vi "Condition _string_FOR_Year.vi"(0 "Select Line 2":string(combo)="ST 1", 1 "connection reference":T1, 2 "Shift":string(combo)="ALL", 3 "BREAKDOWN_STK_HOLD_ID":i32=1, 4 "Found Date":string[](array[string]), 5 "year":string(combo)="ST 1", 7 "error in (no error)":errorcluster) -> (12 "Duration count":string[][](array[string]), 13 "error out":errorcluster, 15 "connection reference 2":T1, 18 "BD Count":string[][](array[string]))   [LabVIEW 2017]
uses:
  <vilib>/addons/database/Connection.llb/Conn ObjectReference.ctl
  <vilib>/addons/database/NI_Database_API.lvlib
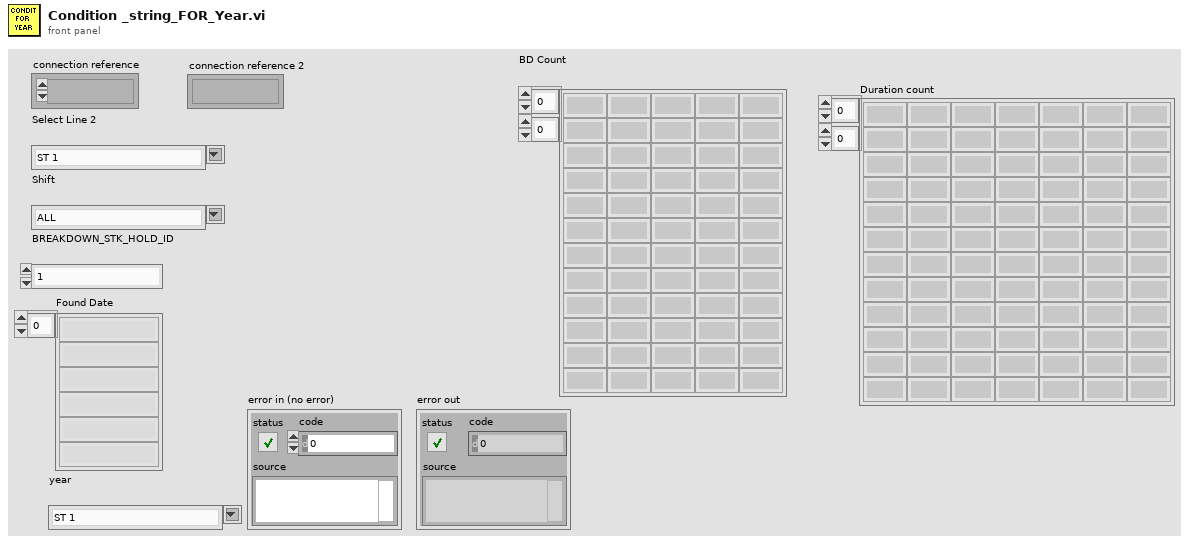
[diagram p1: front panel]
types:
  T1 = typedef "NI_Database_API.lvlib/Conn ObjectReference.ctl" = refnum<k1>
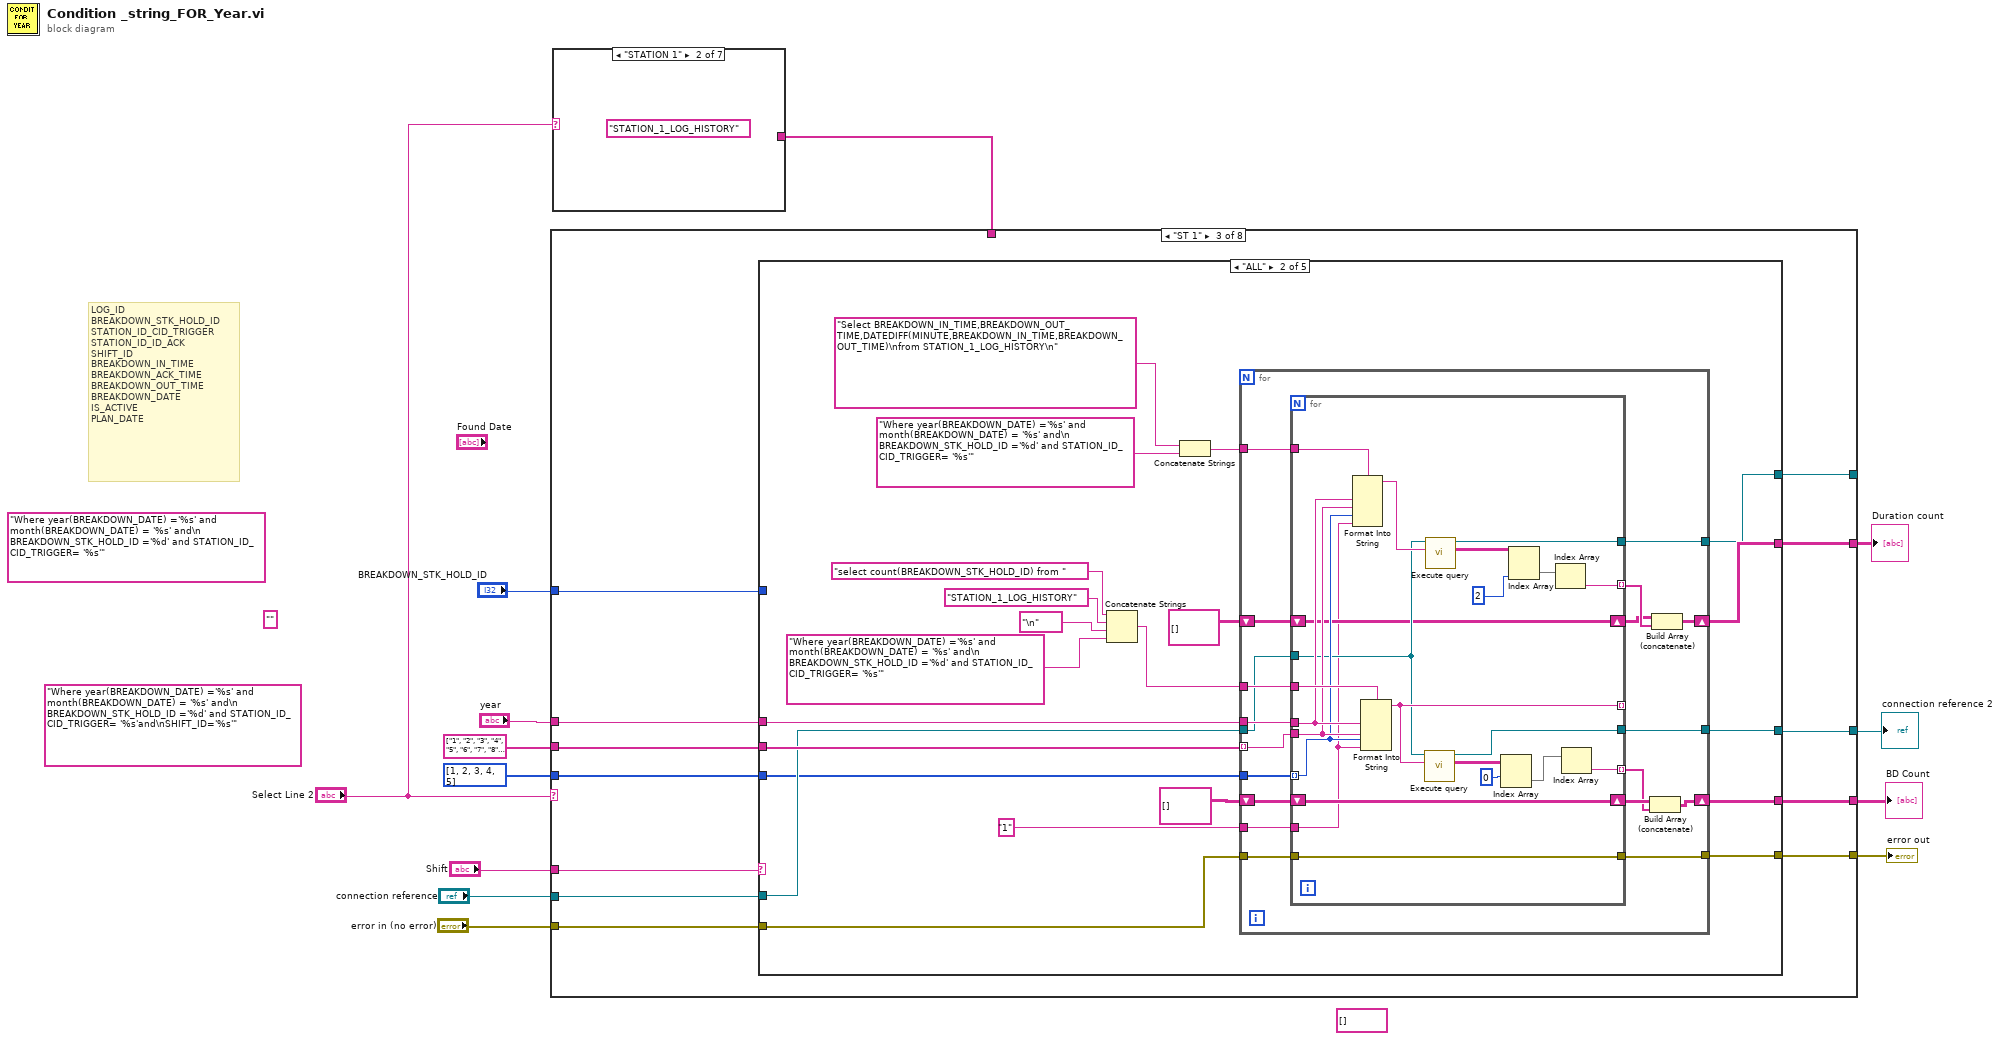
[diagram p0: block diagram]
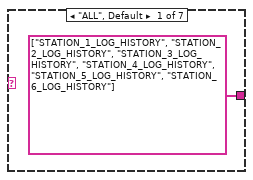
[diagram p2: hidden frame]
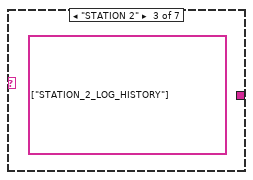
[diagram p3: hidden frame]
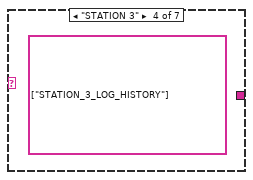
[diagram p4: hidden frame]
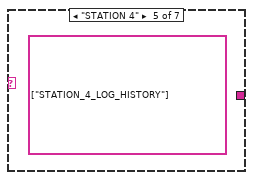
[diagram p5: hidden frame]
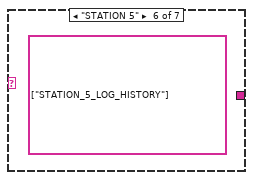
[diagram p6: hidden frame]
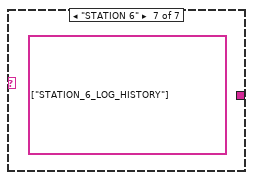
[diagram p7: hidden frame]
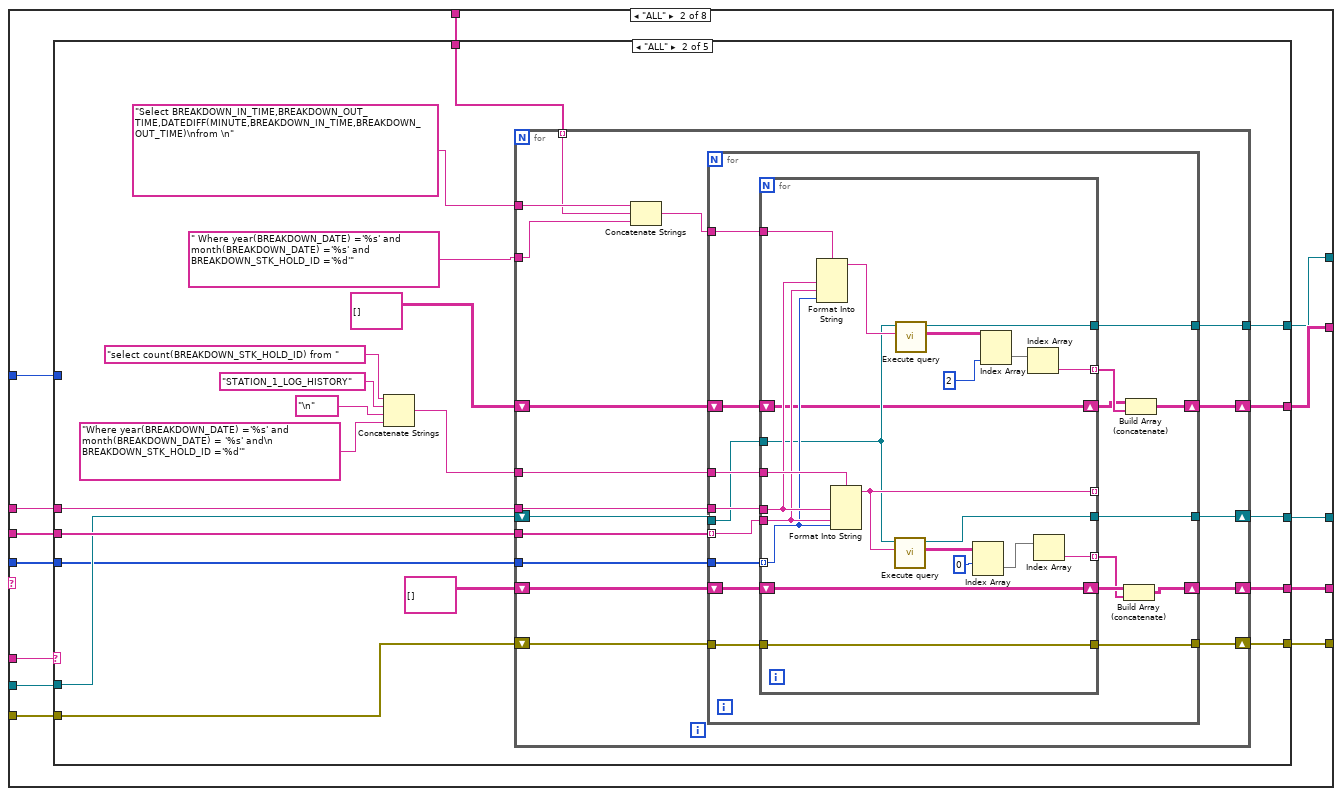
[diagram p9: hidden frame]
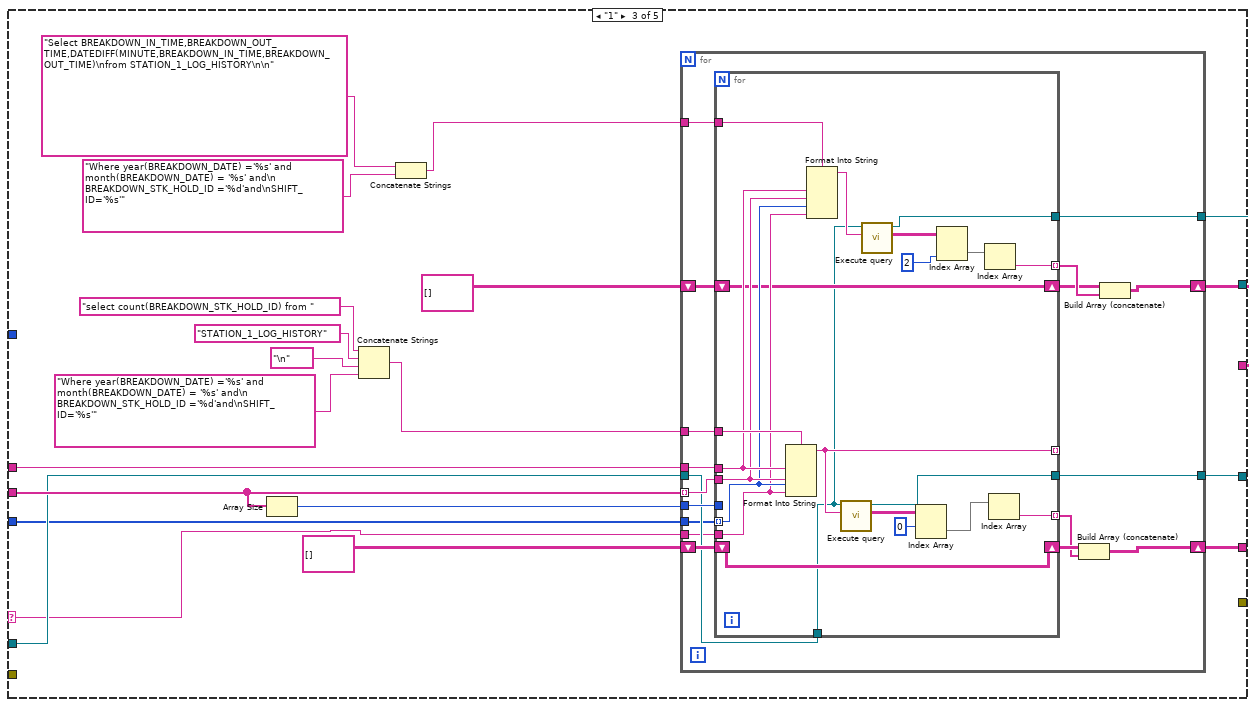
[diagram p11: hidden frame]
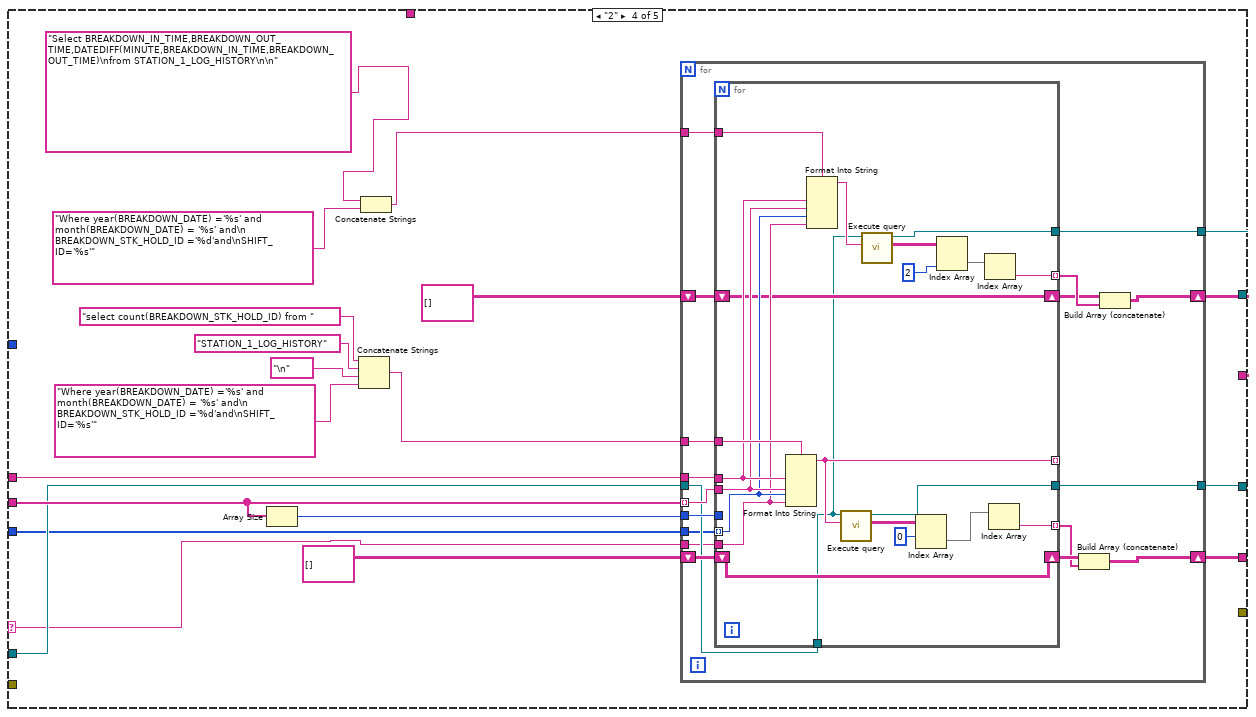
[diagram p12: hidden frame]
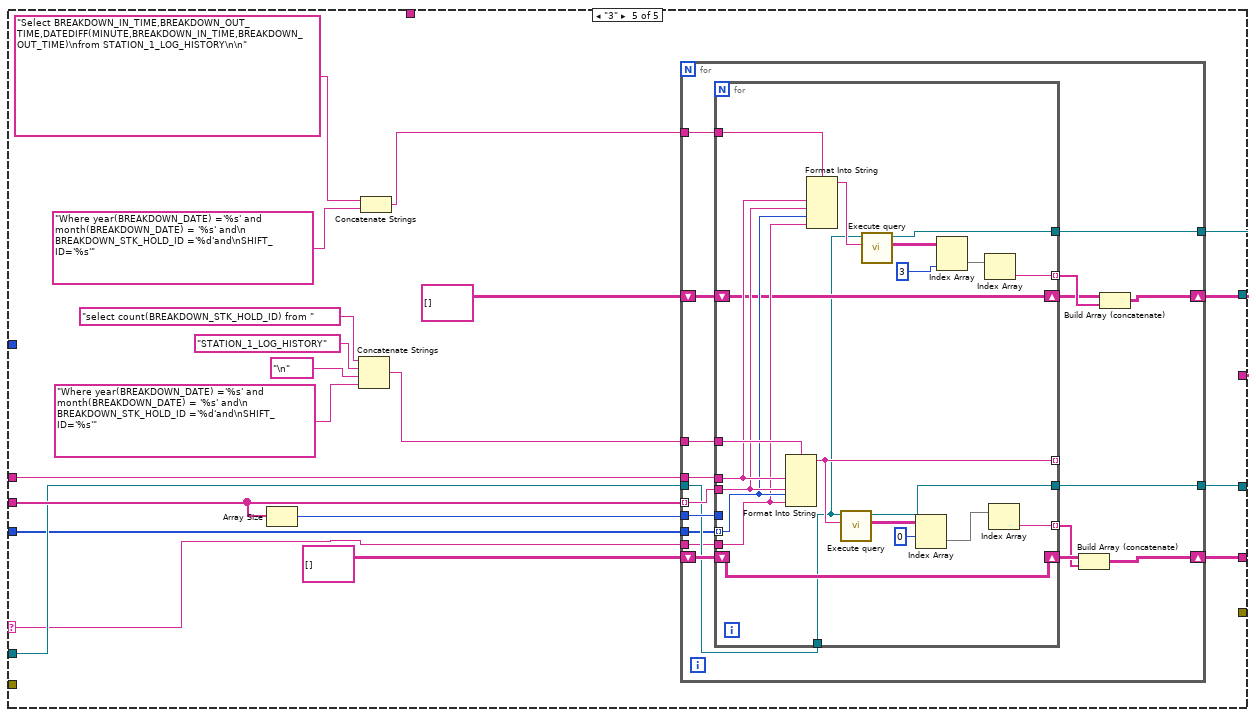
[diagram p13: hidden frame]
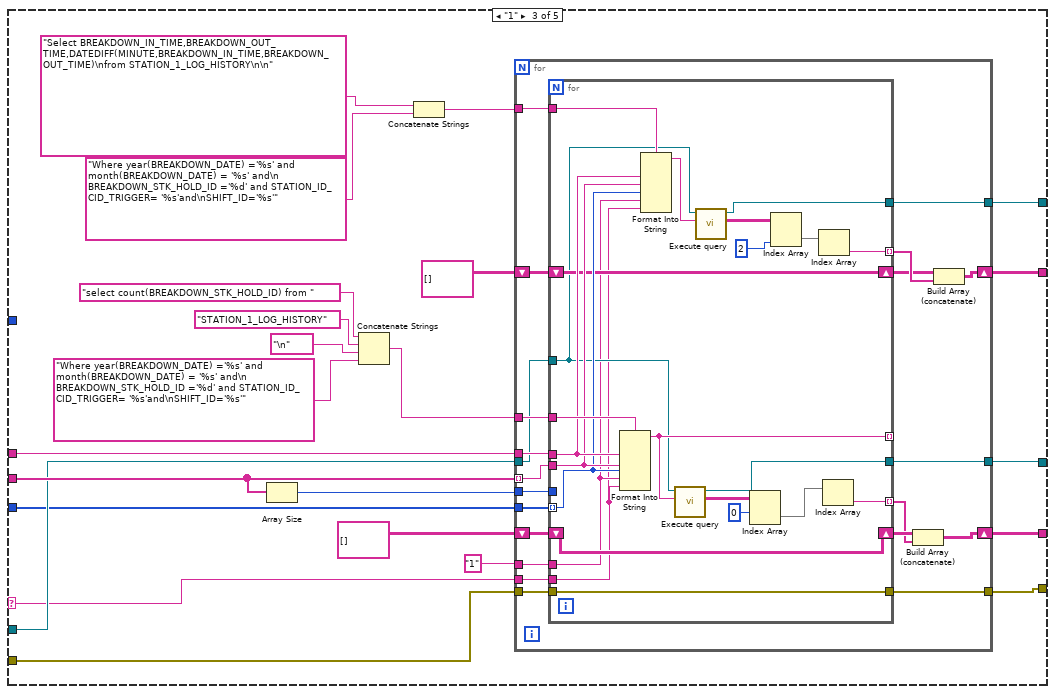
[diagram p15: hidden frame]
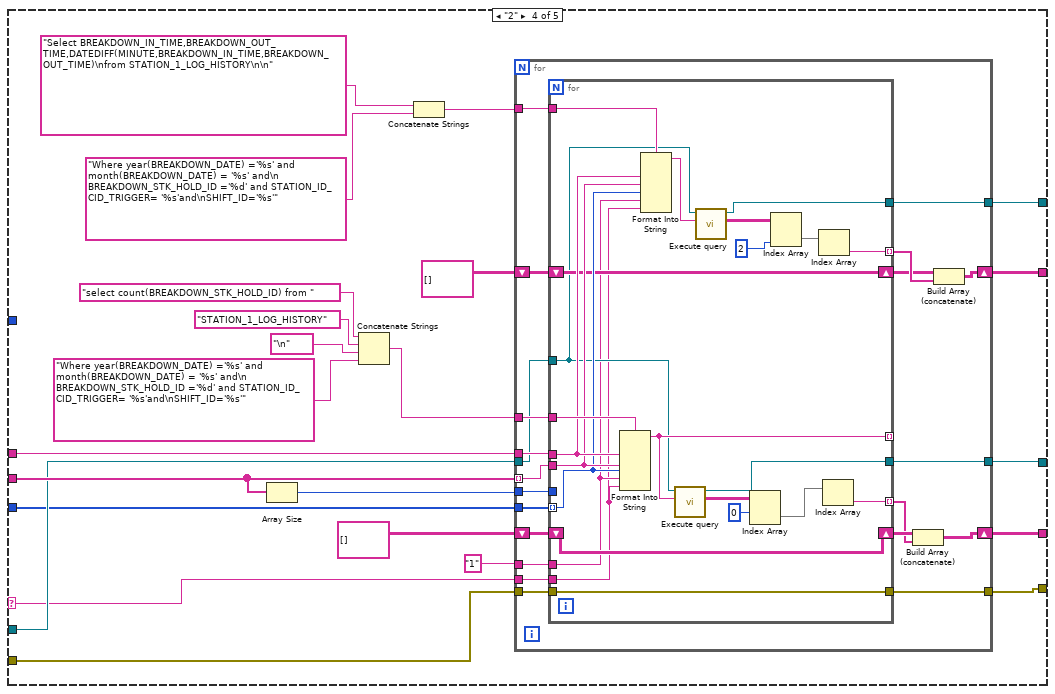
[diagram p16: hidden frame]
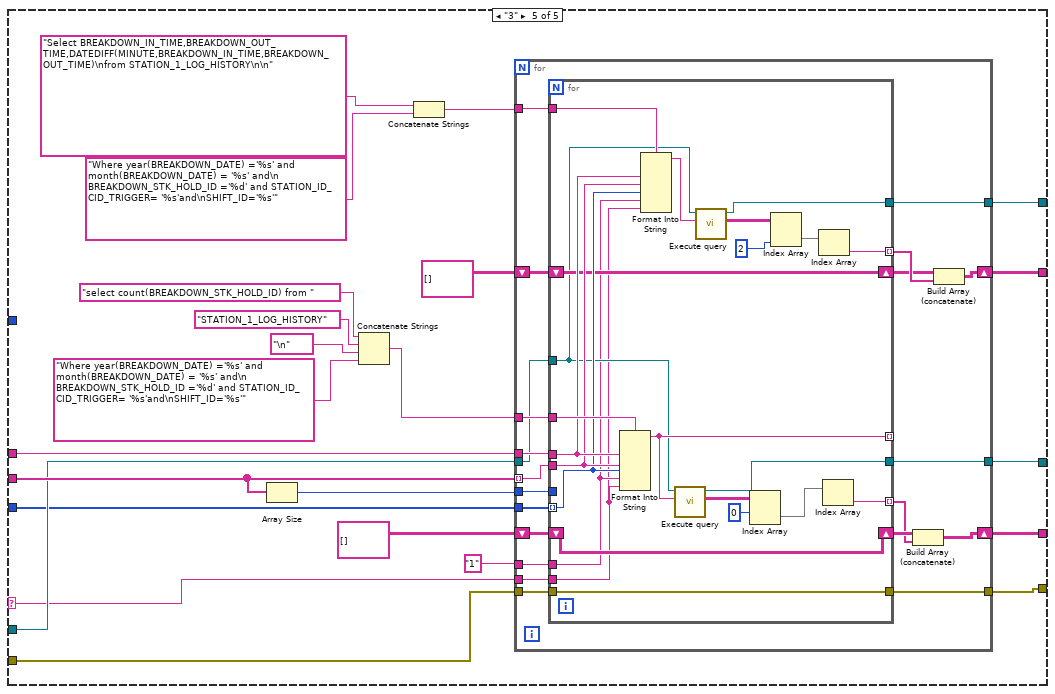
[diagram p17: hidden frame]
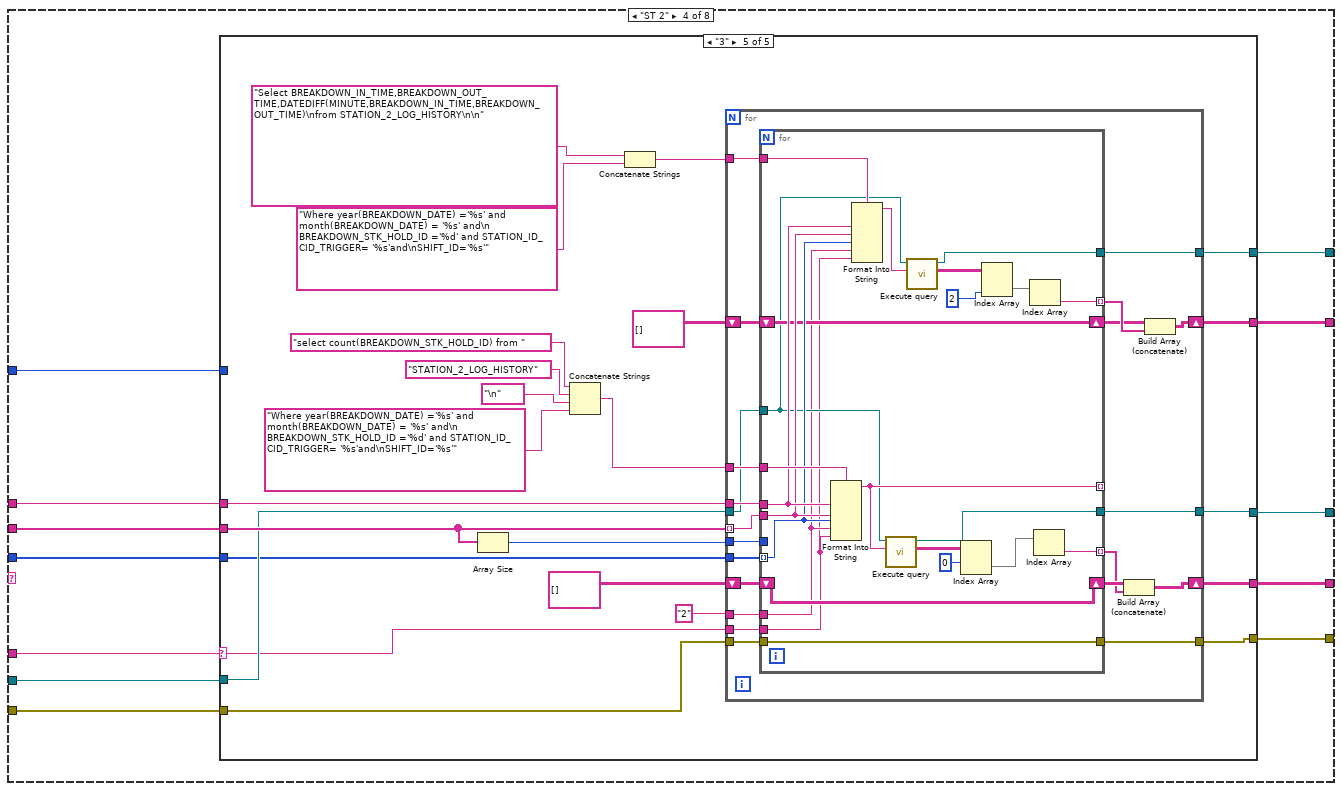
[diagram p18: hidden frame]
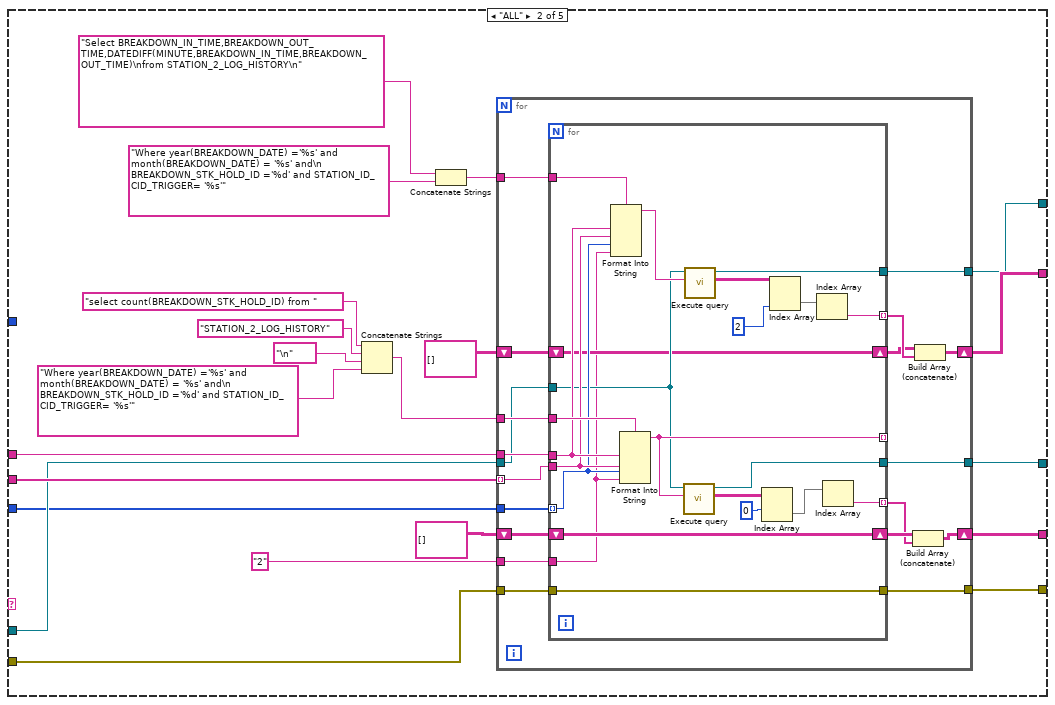
[diagram p20: hidden frame]
diagram:
  (unwired) ""
  (unwired) "Where year(BREAKDOWN_DATE) ='%s' and month(BREAKDOWN_DATE) = '%s' and\n BREAKDOWN_STK_HOLD_ID ='%d' and STATION_ID_CID_TRIGGER= '%s'and\nSHIFT_ID='%s'" ("condition")
  (unwired) "Where year(BREAKDOWN_DATE) ='%s' and month(BREAKDOWN_DATE) = '%s' and\n BREAKDOWN_STK_HOLD_ID ='%d' and STATION_ID_CID_TRIGGER= '%s'" ("condition")
  (unwired) string[] [] ("Output Array")
  # "LOG_ID\nBREAKDOWN_STK_HOLD_ID\nSTATION_ID_CID_TRIGGER\nSTATION_ID_ID_ACK\nSHIFT_ID\nBREAKDOWN_IN_TIME\nBREAKDOWN_ACK_TIME\nBREAKDOWN_OUT_TIME\nBREAKDOWN_DATE\nIS_ACTIVE\nPLAN_DATE"
  n1 = case shown="\"STATION 1\"" "Select Line 2" {
    tunnel: [string[] ["STATION_1_LOG_HISTORY", "STATION_2_LOG_HISTORY", "STATION_3_LOG_HISTORY", "STATION_4_LOG_HISTORY", "STATION_5_LOG_HISTORY", "STATION_6_LOG_HISTORY"] _ _ _ _ _ _] -> w1
    frame "ALL", Default {
    }
    frame "STATION 1" {
      (unwired) "STATION_1_LOG_HISTORY"
    }
    frame "STATION 2" {
      (unwired) string[] ["STATION_2_LOG_HISTORY"]
    }
    frame "STATION 3" {
      (unwired) string[] ["STATION_3_LOG_HISTORY"]
    }
    frame "STATION 4" {
      (unwired) string[] ["STATION_4_LOG_HISTORY"]
    }
    frame "STATION 5" {
      (unwired) string[] ["STATION_5_LOG_HISTORY"]
    }
    frame "STATION 6" {
      (unwired) string[] ["STATION_6_LOG_HISTORY"]
    }
  }
  n2 = case shown="\"ST 1\"" "Select Line 2" {
    tunnel: "Shift" -> [_ w27 w294 w571 w848 w1125 w1402 w1679]
    tunnel: "BREAKDOWN_STK_HOLD_ID" -> [_ w26 w293 w570 w847 w1124 w1401 w1678]
    tunnel: "year" -> [_ w25 w292 w569 w846 w1123 w1400 w1677]
    tunnel: string[] ["1", "2", "3", "4", "5", "6", "7", "8", "9", "10", "11", "12"] -> [_ w24 w291 w568 w845 w1122 w1399 w1676]
    tunnel: [_ w23 w290 w567 w844 w1121 w1398 w1675] -> w9
    tunnel: "connection reference" -> [_ w22 w289 w566 w843 w1120 w1397 w1674]
    tunnel: [_ w21 w288 w565 w842 w1119 w1396 w1673] -> w7
    tunnel: i32[] [1, 2, 3, 4, 5] -> [_ w20 w287 w564 w841 w1118 w1395 w1672]
    tunnel: [_ w19 w286 w563 w840 w1117 w1394 w1671] -> w5
    tunnel: [_ w18 w285 w562 w839 w1116 w1393 w1670] -> _
    tunnel: "error in (no error)" -> [_ w17 w284 w561 w838 w1115 w1392 w1669]
    tunnel: [_ w16 w283 w560 w837 w1114 w1391 w1668] -> w3
    tunnel: w1 -> [_ w15 _ _ _ _ _ _]
    frame "False", Default {
    }
    frame "ALL" {
      n3 = case shown="\"ALL\"" w27 {
        selector: w27 -> [_ _ w112 w171 w230]
        tunnel: w26 -> [_ _ _ _ _]
        tunnel: w25 -> [_ w44 w120 w179 w238]
        tunnel: w24 -> [_ w41 w117 w176 w235]
        tunnel: [_ w45 w121 w180 w239] -> w23
        tunnel: w22 -> [w29 w40 w115 w174 w233]
        tunnel: [w29 w39 w114 w173 w232] -> w21
        tunnel: w20 -> [_ w38 w113 w172 w231]
        tunnel: [_ w36 w109 w167 w226] -> w19
        tunnel: [_ w35 w108 w166 w225] -> w18
        tunnel: w17 -> [w28 w34 _ _ _]
        tunnel: [w28 w33 _ _ _] -> w16
        tunnel: w15 -> [_ w32 _ _ _]
        frame "False", Default {
        }
        frame "ALL" {
          n4 = Concatenate Strings("select count(BREAKDOWN_STK_HOLD_ID) from " ("string"), "STATION_1_LOG_HISTORY" ("table"), "\n" ("string"), "Where year(BREAKDOWN_DATE) ='%s' and month(BREAKDOWN_DATE) = '%s' and\n BREAKDOWN_STK_HOLD_ID ='%d'" ("condition")) -> (w43:string)
          n5 = for {
            tunnel: w44 -> [w65]
            tunnel: w43 -> [w64]
            tunnel: w41 -> [w62]
            tunnel: w38 -> [w59]
            tunnel: [w56] -> w35
            shift-right: [w60] -> w39
            shift-left: w40 -> [w61]
            shift-right: [w54] -> w33
            shift-left: w34 -> [w55]
            tunnel: w32 -> [w51] mode=indexing
            tunnel: "Select BREAKDOWN_IN_TIME,BREAKDOWN_OUT_TIME,DATEDIFF(MINUTE,BREAKDOWN_IN_TIME,BREAKDOWN_OUT_TIME)\nfrom \n" ("string") -> [w53]
            tunnel: " Where year(BREAKDOWN_DATE) ='%s' and month(BREAKDOWN_DATE) ='%s' and BREAKDOWN_STK_HOLD_ID ='%d'" ("condition") -> [w50]
            shift-right: [w57] -> w36
            shift-left: string[][] [] ("Output Array") -> [w58]
            shift-right: [w66] -> w45
            shift-left: string[][] [] ("Output Array") -> [w63]
            n6 = Concatenate Strings(w53, w51, w50) -> (w52:string)
            n7 = for {
              tunnel: w65 -> [w84]
              tunnel: w64 -> [w83]
              tunnel: w62 -> [w81] mode=indexing
              tunnel: w61 -> [w80]
              tunnel: [w79] -> w60
              tunnel: w59 -> [w78]
              shift-right: [w76] -> w66
              shift-left: w63 -> [w82]
              tunnel: w52 -> [w74]
              tunnel: [w73] -> w56
              shift-right: [w69] -> w57
              shift-left: w58 -> [w70]
              tunnel: [w68] -> w54
              tunnel: w55 -> [w67]
              n8 = for {
                tunnel: w83 -> [w105]
                tunnel: w84 -> [w95]
                tunnel: w81 -> [w94]
                tunnel: [w104] -> _ mode=indexing
                tunnel: w80 -> [w92]
                tunnel: [w102] -> w79
                tunnel: w78 -> [w93] mode=indexing
                shift-right: [w103] -> w77
                shift-left: w82 -> [w103]
                tunnel: [w98] -> w75 mode=indexing
                tunnel: w74 -> [w96]
                tunnel: [w89] -> w73
                tunnel: [w88] -> w72 mode=indexing
                shift-right: [w87] -> w71
                shift-left: w70 -> [w87]
                tunnel: [w85] -> w68
                tunnel: w67 -> [w85]
                n9 = Format Into String(format string=w96, w95, w94, w93) -> (resulting string=w97:string)  [unwired: 2 in, 1 out]
                n10 = Format Into String(format string=w105, w95, w94, w93) -> (resulting string=w104:string)  [unwired: 2 in, 1 out]
                n11 = call "Execute query.vi"("String"=w104, "connection reference"=w92) -> ("Table"=w101:string[][], "connection reference 2"=w102:T1)  [unwired: 6 in, 2 out]
                n12 = call "Execute query.vi"("String"=w97, "connection reference"=w92) -> ("Table"=w91:string[][], "connection reference 2"=w89:T1)  [unwired: 6 in, 2 out]
                n13 = Index Array(array=w101, index (row)=0 ("disabled index (col)")) -> (element=w99:string[])  [unwired: 1 in]
                n14 = Index Array(array=w91, index (col)=2 ("disabled index (col)")) -> (element=w90:string[])  [unwired: 1 in]
                n15 = Index Array(array=w90) -> (element=w88:string)  [unwired: 1 in]
                n16 = Index Array(array=w99) -> (element=w98:string)  [unwired: 1 in]
              }
              n17 = Build Array (concatenate)(w77, w75) -> (w76:string[][])
              n18 = Build Array (concatenate)(w71, w72) -> (w69:string[][])
            }
          }
        }
        frame "1" {
          n19 = Array Size(array=w117) -> (size(s)=w116:i32)
          n20 = Concatenate Strings("select count(BREAKDOWN_STK_HOLD_ID) from " ("string"), "STATION_1_LOG_HISTORY" ("table"), "\n" ("string"), "Where year(BREAKDOWN_DATE) ='%s' and month(BREAKDOWN_DATE) = '%s' and\n BREAKDOWN_STK_HOLD_ID ='%d'and\nSHIFT_ID='%s'" ("condition")) -> (w119:string)
          n21 = Concatenate Strings("Select BREAKDOWN_IN_TIME,BREAKDOWN_OUT_TIME,DATEDIFF(MINUTE,BREAKDOWN_IN_TIME,BREAKDOWN_OUT_TIME)\nfrom STATION_1_LOG_HISTORY\n\n" ("string"), "Where year(BREAKDOWN_DATE) ='%s' and month(BREAKDOWN_DATE) = '%s' and\n BREAKDOWN_STK_HOLD_ID ='%d'and\nSHIFT_ID='%s'" ("condition")) -> (w107:string)
          n22 = for {
            tunnel: w120 -> [w143]
            tunnel: w119 -> [w142]
            tunnel: w117 -> [w140] mode=indexing
            tunnel: w116 -> [w139]
            tunnel: w115 -> [w138]
            tunnel: [w137] -> w114
            tunnel: w113 -> [w136]
            shift-right: [w134] -> w121
            shift-left: string[][] [] ("Output Array") -> [w141]
            tunnel: w112 -> [w132]
            tunnel: w107 -> [w131]
            shift-right: [w127] -> w109
            shift-left: string[][] [] ("Output Array") -> [w129]
            tunnel: [w126] -> w108
            n23 = for {
              tunnel: w142 -> [w164]
              tunnel: w143 -> [w152]
              tunnel: w140 -> [w151]
              tunnel: [w163] -> _ mode=indexing
              tunnel: w139 -> [_]
              tunnel: w138 -> [w146]
              tunnel: [w161] -> w137
              tunnel: w136 -> [w150] mode=indexing
              shift-right: [w162] -> w135
              shift-left: w141 -> [w162]
              tunnel: [w158] -> w133 mode=indexing
              tunnel: w132 -> [w149]
              tunnel: w131 -> [w153]
              tunnel: [w148] -> w130 mode=indexing
              shift-right: [w147] -> w128
              shift-left: w129 -> [w147]
              tunnel: [w145] -> w126
              n24 = Format Into String(format string=w164, w152, w151, w150, w149) -> (resulting string=w163:string)  [unwired: 2 in, 1 out]
              n25 = Format Into String(format string=w153, w152, w151, w150, w149) -> (resulting string=w156:string)  [unwired: 2 in, 1 out]
              n26 = call "Execute query.vi"("String"=w163, "connection reference"=w146) -> ("Table"=w157:string[][], "connection reference 2"=w161:T1)  [unwired: 6 in, 2 out]
              n27 = call "Execute query.vi"("String"=w156, "connection reference"=w146) -> ("Table"=w154:string[][], "connection reference 2"=w145:T1)  [unwired: 6 in, 2 out]
              n28 = Index Array(array=w157, index (row)=0 ("disabled index (col)")) -> (element=w159:string[])  [unwired: 1 in]
              n29 = Index Array(array=w154, index (col)=2 ("disabled index (col)")) -> (element=w155:string[])  [unwired: 1 in]
              n30 = Index Array(array=w155) -> (element=w148:string)  [unwired: 1 in]
              n31 = Index Array(array=w159) -> (element=w158:string)  [unwired: 1 in]
            }
            n32 = Build Array (concatenate)(w135, w133) -> (w134:string[][])
            n33 = Build Array (concatenate)(w128, w130) -> (w127:string[][])
          }
        }
        frame "2" {
          n34 = Array Size(array=w176) -> (size(s)=w175:i32)
          n35 = Concatenate Strings("select count(BREAKDOWN_STK_HOLD_ID) from " ("string"), "STATION_1_LOG_HISTORY" ("table"), "\n" ("string"), "Where year(BREAKDOWN_DATE) ='%s' and month(BREAKDOWN_DATE) = '%s' and\n BREAKDOWN_STK_HOLD_ID ='%d'and\nSHIFT_ID='%s'" ("condition")) -> (w178:string)
          n36 = Concatenate Strings("Select BREAKDOWN_IN_TIME,BREAKDOWN_OUT_TIME,DATEDIFF(MINUTE,BREAKDOWN_IN_TIME,BREAKDOWN_OUT_TIME)\nfrom STATION_1_LOG_HISTORY\n\n" ("string"), "Where year(BREAKDOWN_DATE) ='%s' and month(BREAKDOWN_DATE) = '%s' and\n BREAKDOWN_STK_HOLD_ID ='%d'and\nSHIFT_ID='%s'" ("condition")) -> (w169:string)
          n37 = for {
            tunnel: w179 -> [w202]
            tunnel: w178 -> [w201]
            tunnel: w176 -> [w199] mode=indexing
            tunnel: w175 -> [w198]
            tunnel: w174 -> [w197]
            tunnel: [w196] -> w173
            tunnel: w172 -> [w195]
            shift-right: [w193] -> w180
            shift-left: string[][] [] ("Output Array") -> [w200]
            tunnel: w171 -> [w191]
            tunnel: w169 -> [w190]
            shift-right: [w186] -> w167
            shift-left: string[][] [] ("Output Array") -> [w188]
            tunnel: [w185] -> w166
            n38 = for {
              tunnel: w201 -> [w223]
              tunnel: w202 -> [w211]
              tunnel: w199 -> [w210]
              tunnel: [w222] -> _ mode=indexing
              tunnel: w198 -> [_]
              tunnel: w197 -> [w205]
              tunnel: [w220] -> w196
              tunnel: w195 -> [w209] mode=indexing
              shift-right: [w221] -> w194
              shift-left: w200 -> [w221]
              tunnel: [w217] -> w192 mode=indexing
              tunnel: w191 -> [w208]
              tunnel: w190 -> [w212]
              tunnel: [w207] -> w189 mode=indexing
              shift-right: [w206] -> w187
              shift-left: w188 -> [w206]
              tunnel: [w204] -> w185
              n39 = Format Into String(format string=w223, w211, w210, w209, w208) -> (resulting string=w222:string)  [unwired: 2 in, 1 out]
              n40 = Format Into String(format string=w212, w211, w210, w209, w208) -> (resulting string=w215:string)  [unwired: 2 in, 1 out]
              n41 = call "Execute query.vi"("String"=w222, "connection reference"=w205) -> ("Table"=w216:string[][], "connection reference 2"=w220:T1)  [unwired: 6 in, 2 out]
              n42 = call "Execute query.vi"("String"=w215, "connection reference"=w205) -> ("Table"=w213:string[][], "connection reference 2"=w204:T1)  [unwired: 6 in, 2 out]
              n43 = Index Array(array=w216, index (row)=0 ("disabled index (col)")) -> (element=w218:string[])  [unwired: 1 in]
              n44 = Index Array(array=w213, index (col)=2 ("disabled index (col)")) -> (element=w214:string[])  [unwired: 1 in]
              n45 = Index Array(array=w214) -> (element=w207:string)  [unwired: 1 in]
              n46 = Index Array(array=w218) -> (element=w217:string)  [unwired: 1 in]
            }
            n47 = Build Array (concatenate)(w194, w192) -> (w193:string[][])
            n48 = Build Array (concatenate)(w187, w189) -> (w186:string[][])
          }
        }
        frame "3" {
          n49 = Array Size(array=w235) -> (size(s)=w234:i32)
          n50 = Concatenate Strings("select count(BREAKDOWN_STK_HOLD_ID) from " ("string"), "STATION_1_LOG_HISTORY" ("table"), "\n" ("string"), "Where year(BREAKDOWN_DATE) ='%s' and month(BREAKDOWN_DATE) = '%s' and\n BREAKDOWN_STK_HOLD_ID ='%d'and\nSHIFT_ID='%s'" ("condition")) -> (w237:string)
          n51 = Concatenate Strings("Select BREAKDOWN_IN_TIME,BREAKDOWN_OUT_TIME,DATEDIFF(MINUTE,BREAKDOWN_IN_TIME,BREAKDOWN_OUT_TIME)\nfrom STATION_1_LOG_HISTORY\n\n" ("string"), "Where year(BREAKDOWN_DATE) ='%s' and month(BREAKDOWN_DATE) = '%s' and\n BREAKDOWN_STK_HOLD_ID ='%d'and\nSHIFT_ID='%s'" ("condition")) -> (w228:string)
          n52 = for {
            tunnel: w238 -> [w261]
            tunnel: w237 -> [w260]
            tunnel: w235 -> [w258] mode=indexing
            tunnel: w234 -> [w257]
            tunnel: w233 -> [w256]
            tunnel: [w255] -> w232
            tunnel: w231 -> [w254]
            shift-right: [w252] -> w239
            shift-left: string[][] [] ("Output Array") -> [w259]
            tunnel: w230 -> [w250]
            tunnel: w228 -> [w249]
            shift-right: [w245] -> w226
            shift-left: string[][] [] ("Output Array") -> [w247]
            tunnel: [w244] -> w225
            n53 = for {
              tunnel: w260 -> [w282]
              tunnel: w261 -> [w271]
              tunnel: w258 -> [w270]
              tunnel: [w281] -> _ mode=indexing
              tunnel: w257 -> [_]
              tunnel: w256 -> [w263]
              tunnel: [w279] -> w255
              tunnel: w254 -> [w269] mode=indexing
              shift-right: [w280] -> w253
              shift-left: w259 -> [w280]
              tunnel: [w277] -> w251 mode=indexing
              tunnel: w250 -> [w268]
              tunnel: w249 -> [w272]
              tunnel: [w267] -> w248 mode=indexing
              shift-right: [w266] -> w246
              shift-left: w247 -> [w266]
              tunnel: [w264] -> w244
              n54 = Format Into String(format string=w282, w271, w270, w269, w268) -> (resulting string=w281:string)  [unwired: 2 in, 1 out]
              n55 = Format Into String(format string=w272, w271, w270, w269, w268) -> (resulting string=w275:string)  [unwired: 2 in, 1 out]
              n56 = call "Execute query.vi"("String"=w281, "connection reference"=w263) -> ("Table"=w276:string[][], "connection reference 2"=w279:T1)  [unwired: 6 in, 2 out]
              n57 = call "Execute query.vi"("String"=w275, "connection reference"=w263) -> ("Table"=w273:string[][], "connection reference 2"=w264:T1)  [unwired: 6 in, 2 out]
              n58 = Index Array(array=w276, index (row)=0 ("disabled index (col)")) -> (element=w265:string[])  [unwired: 1 in]
              n59 = Index Array(array=w273, index (col)=3 ("disabled index (col)")) -> (element=w274:string[])  [unwired: 1 in]
              n60 = Index Array(array=w274) -> (element=w267:string)  [unwired: 1 in]
              n61 = Index Array(array=w265) -> (element=w277:string)  [unwired: 1 in]
            }
            n62 = Build Array (concatenate)(w253, w251) -> (w252:string[][])
            n63 = Build Array (concatenate)(w246, w248) -> (w245:string[][])
          }
        }
      }
    }
    frame "ST 1" {
      n64 = case shown="\"ALL\"" w294 {
        selector: w294 -> [_ _ w362 w429 w496]
        tunnel: w293 -> [_ _ _ _ _]
        tunnel: w292 -> [_ w313 w377 w444 w511]
        tunnel: w291 -> [_ w310 w374 w441 w508]
        tunnel: [_ w314 w378 w445 w512] -> w290
        tunnel: w289 -> [w296 w309 w372 w439 w506]
        tunnel: [w296 w308 w371 w438 w505] -> w288
        tunnel: w287 -> [_ w307 w370 w437 w504]
        tunnel: [_ w304 w368 w435 w502] -> w286
        tunnel: [_ w303 w367 w434 w501] -> w285
        tunnel: w284 -> [w295 w301 w359 w426 w493]
        tunnel: [w295 w300 w360 w427 w494] -> w283
        frame "False", Default {
        }
        frame "ALL" {
          n65 = Concatenate Strings("select count(BREAKDOWN_STK_HOLD_ID) from " ("string"), "STATION_1_LOG_HISTORY" ("table"), "\n" ("string"), "Where year(BREAKDOWN_DATE) ='%s' and month(BREAKDOWN_DATE) = '%s' and\n BREAKDOWN_STK_HOLD_ID ='%d' and STATION_ID_CID_TRIGGER= '%s'" ("condition")) -> (w312:string)
          n66 = Concatenate Strings("Select BREAKDOWN_IN_TIME,BREAKDOWN_OUT_TIME,DATEDIFF(MINUTE,BREAKDOWN_IN_TIME,BREAKDOWN_OUT_TIME)\nfrom STATION_1_LOG_HISTORY\n" ("string"), "Where year(BREAKDOWN_DATE) ='%s' and month(BREAKDOWN_DATE) = '%s' and\n BREAKDOWN_STK_HOLD_ID ='%d' and STATION_ID_CID_TRIGGER= '%s'" ("condition")) -> (w306:string)
          n67 = for {
            tunnel: w313 -> [w336]
            tunnel: w312 -> [w335]
            tunnel: w310 -> [w333] mode=indexing
            tunnel: w309 -> [w332]
            tunnel: [w331] -> w308
            tunnel: w307 -> [w330]
            shift-right: [w328] -> w314
            shift-left: string[][] [] ("Output Array") -> [w334]
            tunnel: w306 -> [w326]
            tunnel: [w325] -> w303
            shift-right: [w321] -> w304
            shift-left: string[][] [] ("Output Array") -> [w322]
            tunnel: [w320] -> w300
            tunnel: w301 -> [w319]
            tunnel: "1" -> [w318]
            n68 = for {
              tunnel: w335 -> [w358]
              tunnel: w336 -> [w348]
              tunnel: w333 -> [w347]
              tunnel: [w357] -> _ mode=indexing
              tunnel: w332 -> [w345]
              tunnel: [w355] -> w331
              tunnel: w330 -> [w346] mode=indexing
              shift-right: [w356] -> w329
              shift-left: w334 -> [w356]
              tunnel: [w351] -> w327 mode=indexing
              tunnel: w326 -> [w349]
              tunnel: [w342] -> w325
              tunnel: [w341] -> w324 mode=indexing
              shift-right: [w340] -> w323
              shift-left: w322 -> [w340]
              tunnel: [w338] -> w320
              tunnel: w319 -> [w338]
              tunnel: w318 -> [w337]
              n69 = Format Into String(format string=w349, w348, w347, w346, w337) -> (resulting string=w350:string)  [unwired: 2 in, 1 out]
              n70 = Format Into String(format string=w358, w348, w347, w346, w337) -> (resulting string=w357:string)  [unwired: 2 in, 1 out]
              n71 = call "Execute query.vi"("String"=w357, "connection reference"=w345) -> ("Table"=w354:string[][], "connection reference 2"=w355:T1)  [unwired: 6 in, 2 out]
              n72 = call "Execute query.vi"("String"=w350, "connection reference"=w345) -> ("Table"=w344:string[][], "connection reference 2"=w342:T1)  [unwired: 6 in, 2 out]
              n73 = Index Array(array=w354, index (row)=0 ("disabled index (col)")) -> (element=w352:string[])  [unwired: 1 in]
              n74 = Index Array(array=w344, index (col)=2 ("disabled index (col)")) -> (element=w343:string[])  [unwired: 1 in]
              n75 = Index Array(array=w343) -> (element=w341:string)  [unwired: 1 in]
              n76 = Index Array(array=w352) -> (element=w351:string)  [unwired: 1 in]
            }
            n77 = Build Array (concatenate)(w329, w327) -> (w328:string[][])
            n78 = Build Array (concatenate)(w323, w324) -> (w321:string[][])
          }
        }
        frame "1" {
          n79 = Array Size(array=w374) -> (size(s)=w373:i32)
          n80 = Concatenate Strings("select count(BREAKDOWN_STK_HOLD_ID) from " ("string"), "STATION_1_LOG_HISTORY" ("table"), "\n" ("string"), "Where year(BREAKDOWN_DATE) ='%s' and month(BREAKDOWN_DATE) = '%s' and\n BREAKDOWN_STK_HOLD_ID ='%d' and STATION_ID_CID_TRIGGER= '%s'and\nSHIFT_ID='%s'" ("condition")) -> (w376:string)
          n81 = Concatenate Strings("Select BREAKDOWN_IN_TIME,BREAKDOWN_OUT_TIME,DATEDIFF(MINUTE,BREAKDOWN_IN_TIME,BREAKDOWN_OUT_TIME)\nfrom STATION_1_LOG_HISTORY\n\n" ("string"), "Where year(BREAKDOWN_DATE) ='%s' and month(BREAKDOWN_DATE) = '%s' and\n BREAKDOWN_STK_HOLD_ID ='%d' and STATION_ID_CID_TRIGGER= '%s'and\nSHIFT_ID='%s'" ("condition")) -> (w366:string)
          n82 = for {
            tunnel: w377 -> [w402]
            tunnel: w376 -> [w401]
            tunnel: w374 -> [w399] mode=indexing
            tunnel: w373 -> [w398]
            tunnel: w372 -> [w397]
            tunnel: [w396] -> w371
            tunnel: w370 -> [w395]
            shift-right: [w393] -> w378
            shift-left: string[][] [] ("Output Array") -> [w400]
            tunnel: w366 -> [w391]
            shift-right: [w387] -> w368
            shift-left: string[][] [] ("Output Array") -> [w389]
            tunnel: [w386] -> w367
            tunnel: "1" -> [w385]
            tunnel: w362 -> [w384]
            tunnel: [w383] -> w360
            tunnel: w359 -> [w382]
            n83 = for {
              tunnel: w401 -> [w425]
              tunnel: w402 -> [w413]
              tunnel: w399 -> [w412]
              tunnel: [w424] -> _ mode=indexing
              tunnel: w398 -> [_]
              tunnel: w397 -> [w408]
              tunnel: [w422] -> w396
              tunnel: w395 -> [w411] mode=indexing
              shift-right: [w423] -> w394
              shift-left: w400 -> [w423]
              tunnel: [w419] -> w392 mode=indexing
              tunnel: w391 -> [w414]
              tunnel: [w410] -> w390 mode=indexing
              shift-right: [w409] -> w388
              shift-left: w389 -> [w409]
              tunnel: [w407] -> w386
              tunnel: w385 -> [w405]
              tunnel: w384 -> [w404]
              tunnel: [w403] -> w383
              tunnel: w382 -> [w403]
              n84 = Format Into String(format string=w425, w413, w412, w411, w405, w404) -> (resulting string=w424:string)  [unwired: 2 in, 1 out]
              n85 = Format Into String(format string=w414, w413, w412, w411, w405, w404) -> (resulting string=w417:string)  [unwired: 2 in, 1 out]
              n86 = call "Execute query.vi"("String"=w424, "connection reference"=w408) -> ("Table"=w418:string[][], "connection reference 2"=w422:T1)  [unwired: 6 in, 2 out]
              n87 = call "Execute query.vi"("String"=w417, "connection reference"=w408) -> ("Table"=w415:string[][], "connection reference 2"=w407:T1)  [unwired: 6 in, 2 out]
              n88 = Index Array(array=w418, index (row)=0 ("disabled index (col)")) -> (element=w420:string[])  [unwired: 1 in]
              n89 = Index Array(array=w415, index (col)=2 ("disabled index (col)")) -> (element=w416:string[])  [unwired: 1 in]
              n90 = Index Array(array=w416) -> (element=w410:string)  [unwired: 1 in]
              n91 = Index Array(array=w420) -> (element=w419:string)  [unwired: 1 in]
            }
            n92 = Build Array (concatenate)(w394, w392) -> (w393:string[][])
            n93 = Build Array (concatenate)(w388, w390) -> (w387:string[][])
          }
        }
        frame "2" {
          n94 = Array Size(array=w441) -> (size(s)=w440:i32)
          n95 = Concatenate Strings("select count(BREAKDOWN_STK_HOLD_ID) from " ("string"), "STATION_1_LOG_HISTORY" ("table"), "\n" ("string"), "Where year(BREAKDOWN_DATE) ='%s' and month(BREAKDOWN_DATE) = '%s' and\n BREAKDOWN_STK_HOLD_ID ='%d' and STATION_ID_CID_TRIGGER= '%s'and\nSHIFT_ID='%s'" ("condition")) -> (w443:string)
          n96 = Concatenate Strings("Select BREAKDOWN_IN_TIME,BREAKDOWN_OUT_TIME,DATEDIFF(MINUTE,BREAKDOWN_IN_TIME,BREAKDOWN_OUT_TIME)\nfrom STATION_1_LOG_HISTORY\n\n" ("string"), "Where year(BREAKDOWN_DATE) ='%s' and month(BREAKDOWN_DATE) = '%s' and\n BREAKDOWN_STK_HOLD_ID ='%d' and STATION_ID_CID_TRIGGER= '%s'and\nSHIFT_ID='%s'" ("condition")) -> (w433:string)
          n97 = for {
            tunnel: w444 -> [w469]
            tunnel: w443 -> [w468]
            tunnel: w441 -> [w466] mode=indexing
            tunnel: w440 -> [w465]
            tunnel: w439 -> [w464]
            tunnel: [w463] -> w438
            tunnel: w437 -> [w462]
            shift-right: [w460] -> w445
            shift-left: string[][] [] ("Output Array") -> [w467]
            tunnel: w433 -> [w458]
            shift-right: [w454] -> w435
            shift-left: string[][] [] ("Output Array") -> [w456]
            tunnel: [w453] -> w434
            tunnel: "1" -> [w452]
            tunnel: w429 -> [w451]
            tunnel: [w450] -> w427
            tunnel: w426 -> [w449]
            n98 = for {
              tunnel: w468 -> [w492]
              tunnel: w469 -> [w480]
              tunnel: w466 -> [w479]
              tunnel: [w491] -> _ mode=indexing
              tunnel: w465 -> [_]
              tunnel: w464 -> [w475]
              tunnel: [w489] -> w463
              tunnel: w462 -> [w478] mode=indexing
              shift-right: [w490] -> w461
              shift-left: w467 -> [w490]
              tunnel: [w486] -> w459 mode=indexing
              tunnel: w458 -> [w481]
              tunnel: [w477] -> w457 mode=indexing
              shift-right: [w476] -> w455
              shift-left: w456 -> [w476]
              tunnel: [w474] -> w453
              tunnel: w452 -> [w472]
              tunnel: w451 -> [w471]
              tunnel: [w470] -> w450
              tunnel: w449 -> [w470]
              n99 = Format Into String(format string=w492, w480, w479, w478, w472, w471) -> (resulting string=w491:string)  [unwired: 2 in, 1 out]
              n100 = Format Into String(format string=w481, w480, w479, w478, w472, w471) -> (resulting string=w484:string)  [unwired: 2 in, 1 out]
              n101 = call "Execute query.vi"("String"=w491, "connection reference"=w475) -> ("Table"=w485:string[][], "connection reference 2"=w489:T1)  [unwired: 6 in, 2 out]
              n102 = call "Execute query.vi"("String"=w484, "connection reference"=w475) -> ("Table"=w482:string[][], "connection reference 2"=w474:T1)  [unwired: 6 in, 2 out]
              n103 = Index Array(array=w485, index (row)=0 ("disabled index (col)")) -> (element=w487:string[])  [unwired: 1 in]
              n104 = Index Array(array=w482, index (col)=2 ("disabled index (col)")) -> (element=w483:string[])  [unwired: 1 in]
              n105 = Index Array(array=w483) -> (element=w477:string)  [unwired: 1 in]
              n106 = Index Array(array=w487) -> (element=w486:string)  [unwired: 1 in]
            }
            n107 = Build Array (concatenate)(w461, w459) -> (w460:string[][])
            n108 = Build Array (concatenate)(w455, w457) -> (w454:string[][])
          }
        }
        frame "3" {
          n109 = Array Size(array=w508) -> (size(s)=w507:i32)
          n110 = Concatenate Strings("select count(BREAKDOWN_STK_HOLD_ID) from " ("string"), "STATION_1_LOG_HISTORY" ("table"), "\n" ("string"), "Where year(BREAKDOWN_DATE) ='%s' and month(BREAKDOWN_DATE) = '%s' and\n BREAKDOWN_STK_HOLD_ID ='%d' and STATION_ID_CID_TRIGGER= '%s'and\nSHIFT_ID='%s'" ("condition")) -> (w510:string)
          n111 = Concatenate Strings("Select BREAKDOWN_IN_TIME,BREAKDOWN_OUT_TIME,DATEDIFF(MINUTE,BREAKDOWN_IN_TIME,BREAKDOWN_OUT_TIME)\nfrom STATION_1_LOG_HISTORY\n\n" ("string"), "Where year(BREAKDOWN_DATE) ='%s' and month(BREAKDOWN_DATE) = '%s' and\n BREAKDOWN_STK_HOLD_ID ='%d' and STATION_ID_CID_TRIGGER= '%s'and\nSHIFT_ID='%s'" ("condition")) -> (w500:string)
          n112 = for {
            tunnel: w511 -> [w536]
            tunnel: w510 -> [w535]
            tunnel: w508 -> [w533] mode=indexing
            tunnel: w507 -> [w532]
            tunnel: w506 -> [w531]
            tunnel: [w530] -> w505
            tunnel: w504 -> [w529]
            shift-right: [w527] -> w512
            shift-left: string[][] [] ("Output Array") -> [w534]
            tunnel: w500 -> [w525]
            shift-right: [w521] -> w502
            shift-left: string[][] [] ("Output Array") -> [w523]
            tunnel: [w520] -> w501
            tunnel: "1" -> [w519]
            tunnel: w496 -> [w518]
            tunnel: [w517] -> w494
            tunnel: w493 -> [w516]
            n113 = for {
              tunnel: w535 -> [w559]
              tunnel: w536 -> [w547]
              tunnel: w533 -> [w546]
              tunnel: [w558] -> _ mode=indexing
              tunnel: w532 -> [_]
              tunnel: w531 -> [w542]
              tunnel: [w556] -> w530
              tunnel: w529 -> [w545] mode=indexing
              shift-right: [w557] -> w528
              shift-left: w534 -> [w557]
              tunnel: [w553] -> w526 mode=indexing
              tunnel: w525 -> [w548]
              tunnel: [w544] -> w524 mode=indexing
              shift-right: [w543] -> w522
              shift-left: w523 -> [w543]
              tunnel: [w541] -> w520
              tunnel: w519 -> [w539]
              tunnel: w518 -> [w538]
              tunnel: [w537] -> w517
              tunnel: w516 -> [w537]
              n114 = Format Into String(format string=w559, w547, w546, w545, w539, w538) -> (resulting string=w558:string)  [unwired: 2 in, 1 out]
              n115 = Format Into String(format string=w548, w547, w546, w545, w539, w538) -> (resulting string=w551:string)  [unwired: 2 in, 1 out]
              n116 = call "Execute query.vi"("String"=w558, "connection reference"=w542) -> ("Table"=w552:string[][], "connection reference 2"=w556:T1)  [unwired: 6 in, 2 out]
              n117 = call "Execute query.vi"("String"=w551, "connection reference"=w542) -> ("Table"=w549:string[][], "connection reference 2"=w541:T1)  [unwired: 6 in, 2 out]
              n118 = Index Array(array=w552, index (row)=0 ("disabled index (col)")) -> (element=w554:string[])  [unwired: 1 in]
              n119 = Index Array(array=w549, index (col)=2 ("disabled index (col)")) -> (element=w550:string[])  [unwired: 1 in]
              n120 = Index Array(array=w550) -> (element=w544:string)  [unwired: 1 in]
              n121 = Index Array(array=w554) -> (element=w553:string)  [unwired: 1 in]
            }
            n122 = Build Array (concatenate)(w528, w526) -> (w527:string[][])
            n123 = Build Array (concatenate)(w522, w524) -> (w521:string[][])
          }
        }
      }
    }
    frame "ST 2" {
      n124 = case shown="\"3\"" w571 {
        selector: w571 -> [_ _ w639 w706 w773]
        tunnel: w570 -> [_ _ _ _ _]
        tunnel: w569 -> [_ w590 w654 w721 w788]
        tunnel: w568 -> [_ w587 w651 w718 w785]
        tunnel: [_ w591 w655 w722 w789] -> w567
        tunnel: w566 -> [w573 w586 w649 w716 w783]
        tunnel: [w573 w585 w648 w715 w782] -> w565
        tunnel: w564 -> [_ w584 w647 w714 w781]
        tunnel: [_ w581 w645 w712 w779] -> w563
        tunnel: [_ w580 w644 w711 w778] -> w562
        tunnel: w561 -> [w572 w578 w636 w703 w770]
        tunnel: [w572 w577 w637 w704 w771] -> w560
        frame "False", Default {
        }
        frame "ALL" {
          n125 = Concatenate Strings("select count(BREAKDOWN_STK_HOLD_ID) from " ("string"), "STATION_2_LOG_HISTORY" ("table"), "\n" ("string"), "Where year(BREAKDOWN_DATE) ='%s' and month(BREAKDOWN_DATE) = '%s' and\n BREAKDOWN_STK_HOLD_ID ='%d' and STATION_ID_CID_TRIGGER= '%s'" ("condition")) -> (w589:string)
          n126 = Concatenate Strings("Select BREAKDOWN_IN_TIME,BREAKDOWN_OUT_TIME,DATEDIFF(MINUTE,BREAKDOWN_IN_TIME,BREAKDOWN_OUT_TIME)\nfrom STATION_2_LOG_HISTORY\n" ("string"), "Where year(BREAKDOWN_DATE) ='%s' and month(BREAKDOWN_DATE) = '%s' and\n BREAKDOWN_STK_HOLD_ID ='%d' and STATION_ID_CID_TRIGGER= '%s'" ("condition")) -> (w583:string)
          n127 = for {
            tunnel: w590 -> [w613]
            tunnel: w589 -> [w612]
            tunnel: w587 -> [w610] mode=indexing
            tunnel: w586 -> [w609]
            tunnel: [w608] -> w585
            tunnel: w584 -> [w607]
            shift-right: [w605] -> w591
            shift-left: string[][] [] ("Output Array") -> [w611]
            tunnel: w583 -> [w603]
            tunnel: [w602] -> w580
            shift-right: [w598] -> w581
            shift-left: string[][] [] ("Output Array") -> [w599]
            tunnel: [w597] -> w577
            tunnel: w578 -> [w596]
            tunnel: "2" -> [w595]
            n128 = for {
              tunnel: w612 -> [w635]
              tunnel: w613 -> [w625]
              tunnel: w610 -> [w624]
              tunnel: [w634] -> _ mode=indexing
              tunnel: w609 -> [w622]
              tunnel: [w632] -> w608
              tunnel: w607 -> [w623] mode=indexing
              shift-right: [w633] -> w606
              shift-left: w611 -> [w633]
              tunnel: [w628] -> w604 mode=indexing
              tunnel: w603 -> [w626]
              tunnel: [w619] -> w602
              tunnel: [w618] -> w601 mode=indexing
              shift-right: [w617] -> w600
              shift-left: w599 -> [w617]
              tunnel: [w615] -> w597
              tunnel: w596 -> [w615]
              tunnel: w595 -> [w614]
              n129 = Format Into String(format string=w626, w625, w624, w623, w614) -> (resulting string=w627:string)  [unwired: 2 in, 1 out]
              n130 = Format Into String(format string=w635, w625, w624, w623, w614) -> (resulting string=w634:string)  [unwired: 2 in, 1 out]
              n131 = call "Execute query.vi"("String"=w634, "connection reference"=w622) -> ("Table"=w631:string[][], "connection reference 2"=w632:T1)  [unwired: 6 in, 2 out]
              n132 = call "Execute query.vi"("String"=w627, "connection reference"=w622) -> ("Table"=w621:string[][], "connection reference 2"=w619:T1)  [unwired: 6 in, 2 out]
              n133 = Index Array(array=w631, index (row)=0 ("disabled index (col)")) -> (element=w629:string[])  [unwired: 1 in]
              n134 = Index Array(array=w621, index (col)=2 ("disabled index (col)")) -> (element=w620:string[])  [unwired: 1 in]
              n135 = Index Array(array=w620) -> (element=w618:string)  [unwired: 1 in]
              n136 = Index Array(array=w629) -> (element=w628:string)  [unwired: 1 in]
            }
            n137 = Build Array (concatenate)(w606, w604) -> (w605:string[][])
            n138 = Build Array (concatenate)(w600, w601) -> (w598:string[][])
          }
        }
        frame "1" {
          n139 = Array Size(array=w651) -> (size(s)=w650:i32)
          n140 = Concatenate Strings("select count(BREAKDOWN_STK_HOLD_ID) from " ("string"), "STATION_2_LOG_HISTORY" ("table"), "\n" ("string"), "Where year(BREAKDOWN_DATE) ='%s' and month(BREAKDOWN_DATE) = '%s' and\n BREAKDOWN_STK_HOLD_ID ='%d' and STATION_ID_CID_TRIGGER= '%s'and\nSHIFT_ID='%s'" ("condition")) -> (w653:string)
          n141 = Concatenate Strings("Select BREAKDOWN_IN_TIME,BREAKDOWN_OUT_TIME,DATEDIFF(MINUTE,BREAKDOWN_IN_TIME,BREAKDOWN_OUT_TIME)\nfrom STATION_2_LOG_HISTORY\n\n" ("string"), "Where year(BREAKDOWN_DATE) ='%s' and month(BREAKDOWN_DATE) = '%s' and\n BREAKDOWN_STK_HOLD_ID ='%d' and STATION_ID_CID_TRIGGER= '%s'and\nSHIFT_ID='%s'" ("condition")) -> (w643:string)
          n142 = for {
            tunnel: w654 -> [w679]
            tunnel: w653 -> [w678]
            tunnel: w651 -> [w676] mode=indexing
            tunnel: w650 -> [w675]
            tunnel: w649 -> [w674]
            tunnel: [w673] -> w648
            tunnel: w647 -> [w672]
            shift-right: [w670] -> w655
            shift-left: string[][] [] ("Output Array") -> [w677]
            tunnel: w643 -> [w668]
            shift-right: [w664] -> w645
            shift-left: string[][] [] ("Output Array") -> [w666]
            tunnel: [w663] -> w644
            tunnel: "2" -> [w662]
            tunnel: w639 -> [w661]
            tunnel: [w660] -> w637
            tunnel: w636 -> [w659]
            n143 = for {
              tunnel: w678 -> [w702]
              tunnel: w679 -> [w690]
              tunnel: w676 -> [w689]
              tunnel: [w701] -> _ mode=indexing
              tunnel: w675 -> [_]
              tunnel: w674 -> [w685]
              tunnel: [w699] -> w673
              tunnel: w672 -> [w688] mode=indexing
              shift-right: [w700] -> w671
              shift-left: w677 -> [w700]
              tunnel: [w696] -> w669 mode=indexing
              tunnel: w668 -> [w691]
              tunnel: [w687] -> w667 mode=indexing
              shift-right: [w686] -> w665
              shift-left: w666 -> [w686]
              tunnel: [w684] -> w663
              tunnel: w662 -> [w682]
              tunnel: w661 -> [w681]
              tunnel: [w680] -> w660
              tunnel: w659 -> [w680]
              n144 = Format Into String(format string=w702, w690, w689, w688, w682, w681) -> (resulting string=w701:string)  [unwired: 2 in, 1 out]
              n145 = Format Into String(format string=w691, w690, w689, w688, w682, w681) -> (resulting string=w694:string)  [unwired: 2 in, 1 out]
              n146 = call "Execute query.vi"("String"=w701, "connection reference"=w685) -> ("Table"=w695:string[][], "connection reference 2"=w699:T1)  [unwired: 6 in, 2 out]
              n147 = call "Execute query.vi"("String"=w694, "connection reference"=w685) -> ("Table"=w692:string[][], "connection reference 2"=w684:T1)  [unwired: 6 in, 2 out]
              n148 = Index Array(array=w695, index (row)=0 ("disabled index (col)")) -> (element=w697:string[])  [unwired: 1 in]
              n149 = Index Array(array=w692, index (col)=2 ("disabled index (col)")) -> (element=w693:string[])  [unwired: 1 in]
              n150 = Index Array(array=w693) -> (element=w687:string)  [unwired: 1 in]
              n151 = Index Array(array=w697) -> (element=w696:string)  [unwired: 1 in]
            }
            n152 = Build Array (concatenate)(w671, w669) -> (w670:string[][])
            n153 = Build Array (concatenate)(w665, w667) -> (w664:string[][])
          }
        }
        frame "2" {
          n154 = Array Size(array=w718) -> (size(s)=w717:i32)
          n155 = Concatenate Strings("select count(BREAKDOWN_STK_HOLD_ID) from " ("string"), "STATION_2_LOG_HISTORY" ("table"), "\n" ("string"), "Where year(BREAKDOWN_DATE) ='%s' and month(BREAKDOWN_DATE) = '%s' and\n BREAKDOWN_STK_HOLD_ID ='%d' and STATION_ID_CID_TRIGGER= '%s'and\nSHIFT_ID='%s'" ("condition")) -> (w720:string)
          n156 = Concatenate Strings("Select BREAKDOWN_IN_TIME,BREAKDOWN_OUT_TIME,DATEDIFF(MINUTE,BREAKDOWN_IN_TIME,BREAKDOWN_OUT_TIME)\nfrom STATION_2_LOG_HISTORY\n\n" ("string"), "Where year(BREAKDOWN_DATE) ='%s' and month(BREAKDOWN_DATE) = '%s' and\n BREAKDOWN_STK_HOLD_ID ='%d' and STATION_ID_CID_TRIGGER= '%s'and\nSHIFT_ID='%s'" ("condition")) -> (w710:string)
          n157 = for {
            tunnel: w721 -> [w746]
            tunnel: w720 -> [w745]
            tunnel: w718 -> [w743] mode=indexing
            tunnel: w717 -> [w742]
            tunnel: w716 -> [w741]
            tunnel: [w740] -> w715
            tunnel: w714 -> [w739]
            shift-right: [w737] -> w722
            shift-left: string[][] [] ("Output Array") -> [w744]
            tunnel: w710 -> [w735]
            shift-right: [w731] -> w712
            shift-left: string[][] [] ("Output Array") -> [w733]
            tunnel: [w730] -> w711
            tunnel: "2" -> [w729]
            tunnel: w706 -> [w728]
            tunnel: [w727] -> w704
            tunnel: w703 -> [w726]
            n158 = for {
              tunnel: w745 -> [w769]
              tunnel: w746 -> [w757]
              tunnel: w743 -> [w756]
              tunnel: [w768] -> _ mode=indexing
              tunnel: w742 -> [_]
              tunnel: w741 -> [w752]
              tunnel: [w766] -> w740
              tunnel: w739 -> [w755] mode=indexing
              shift-right: [w767] -> w738
              shift-left: w744 -> [w767]
              tunnel: [w763] -> w736 mode=indexing
              tunnel: w735 -> [w758]
              tunnel: [w754] -> w734 mode=indexing
              shift-right: [w753] -> w732
              shift-left: w733 -> [w753]
              tunnel: [w751] -> w730
              tunnel: w729 -> [w749]
              tunnel: w728 -> [w748]
              tunnel: [w747] -> w727
              tunnel: w726 -> [w747]
              n159 = Format Into String(format string=w769, w757, w756, w755, w749, w748) -> (resulting string=w768:string)  [unwired: 2 in, 1 out]
              n160 = Format Into String(format string=w758, w757, w756, w755, w749, w748) -> (resulting string=w761:string)  [unwired: 2 in, 1 out]
              n161 = call "Execute query.vi"("String"=w768, "connection reference"=w752) -> ("Table"=w762:string[][], "connection reference 2"=w766:T1)  [unwired: 6 in, 2 out]
              n162 = call "Execute query.vi"("String"=w761, "connection reference"=w752) -> ("Table"=w759:string[][], "connection reference 2"=w751:T1)  [unwired: 6 in, 2 out]
              n163 = Index Array(array=w762, index (row)=0 ("disabled index (col)")) -> (element=w764:string[])  [unwired: 1 in]
              n164 = Index Array(array=w759, index (col)=2 ("disabled index (col)")) -> (element=w760:string[])  [unwired: 1 in]
              n165 = Index Array(array=w760) -> (element=w754:string)  [unwired: 1 in]
              n166 = Index Array(array=w764) -> (element=w763:string)  [unwired: 1 in]
            }
            n167 = Build Array (concatenate)(w738, w736) -> (w737:string[][])
            n168 = Build Array (concatenate)(w732, w734) -> (w731:string[][])
          }
        }
        frame "3" {
          n169 = Array Size(array=w785) -> (size(s)=w784:i32)
          n170 = Concatenate Strings("select count(BREAKDOWN_STK_HOLD_ID) from " ("string"), "STATION_2_LOG_HISTORY" ("table"), "\n" ("string"), "Where year(BREAKDOWN_DATE) ='%s' and month(BREAKDOWN_DATE) = '%s' and\n BREAKDOWN_STK_HOLD_ID ='%d' and STATION_ID_CID_TRIGGER= '%s'and\nSHIFT_ID='%s'" ("condition")) -> (w787:string)
          n171 = Concatenate Strings("Select BREAKDOWN_IN_TIME,BREAKDOWN_OUT_TIME,DATEDIFF(MINUTE,BREAKDOWN_IN_TIME,BREAKDOWN_OUT_TIME)\nfrom STATION_2_LOG_HISTORY\n\n" ("string"), "Where year(BREAKDOWN_DATE) ='%s' and month(BREAKDOWN_DATE) = '%s' and\n BREAKDOWN_STK_HOLD_ID ='%d' and STATION_ID_CID_TRIGGER= '%s'and\nSHIFT_ID='%s'" ("condition")) -> (w777:string)
          n172 = for {
            tunnel: w788 -> [w813]
            tunnel: w787 -> [w812]
            tunnel: w785 -> [w810] mode=indexing
            tunnel: w784 -> [w809]
            tunnel: w783 -> [w808]
            tunnel: [w807] -> w782
            tunnel: w781 -> [w806]
            shift-right: [w804] -> w789
            shift-left: string[][] [] ("Output Array") -> [w811]
            tunnel: w777 -> [w802]
            shift-right: [w798] -> w779
            shift-left: string[][] [] ("Output Array") -> [w800]
            tunnel: [w797] -> w778
            tunnel: "2" -> [w796]
            tunnel: w773 -> [w795]
            tunnel: [w794] -> w771
            tunnel: w770 -> [w793]
            n173 = for {
              tunnel: w812 -> [w836]
              tunnel: w813 -> [w824]
              tunnel: w810 -> [w823]
              tunnel: [w835] -> _ mode=indexing
              tunnel: w809 -> [_]
              tunnel: w808 -> [w819]
              tunnel: [w833] -> w807
              tunnel: w806 -> [w822] mode=indexing
              shift-right: [w834] -> w805
              shift-left: w811 -> [w834]
              tunnel: [w830] -> w803 mode=indexing
              tunnel: w802 -> [w825]
              tunnel: [w821] -> w801 mode=indexing
              shift-right: [w820] -> w799
              shift-left: w800 -> [w820]
              tunnel: [w818] -> w797
              tunnel: w796 -> [w816]
              tunnel: w795 -> [w815]
              tunnel: [w814] -> w794
              tunnel: w793 -> [w814]
              n174 = Format Into String(format string=w836, w824, w823, w822, w816, w815) -> (resulting string=w835:string)  [unwired: 2 in, 1 out]
              n175 = Format Into String(format string=w825, w824, w823, w822, w816, w815) -> (resulting string=w828:string)  [unwired: 2 in, 1 out]
              n176 = call "Execute query.vi"("String"=w835, "connection reference"=w819) -> ("Table"=w829:string[][], "connection reference 2"=w833:T1)  [unwired: 6 in, 2 out]
              n177 = call "Execute query.vi"("String"=w828, "connection reference"=w819) -> ("Table"=w826:string[][], "connection reference 2"=w818:T1)  [unwired: 6 in, 2 out]
              n178 = Index Array(array=w829, index (row)=0 ("disabled index (col)")) -> (element=w831:string[])  [unwired: 1 in]
              n179 = Index Array(array=w826, index (col)=2 ("disabled index (col)")) -> (element=w827:string[])  [unwired: 1 in]
              n180 = Index Array(array=w827) -> (element=w821:string)  [unwired: 1 in]
              n181 = Index Array(array=w831) -> (element=w830:string)  [unwired: 1 in]
            }
            n182 = Build Array (concatenate)(w805, w803) -> (w804:string[][])
            n183 = Build Array (concatenate)(w799, w801) -> (w798:string[][])
          }
        }
      }
    }
    frame "ST 3" {
      n184 = case shown="\"ALL\"" w848 {
        selector: w848 -> [_ _ w916 w983 w1050]
        tunnel: w847 -> [_ _ _ _ _]
        tunnel: w846 -> [_ w867 w931 w998 w1065]
        tunnel: w845 -> [_ w864 w928 w995 w1062]
        tunnel: [_ w868 w932 w999 w1066] -> w844
        tunnel: w843 -> [w850 w863 w926 w993 w1060]
        tunnel: [w850 w862 w925 w992 w1059] -> w842
        tunnel: w841 -> [_ w861 w924 w991 w1058]
        tunnel: [_ w858 w922 w989 w1056] -> w840
        tunnel: [_ w857 w921 w988 w1055] -> w839
        tunnel: w838 -> [w849 w855 w913 w980 w1047]
        tunnel: [w849 w854 w914 w981 w1048] -> w837
        frame "False", Default {
        }
        frame "ALL" {
          n185 = Concatenate Strings("select count(BREAKDOWN_STK_HOLD_ID) from " ("string"), "STATION_3_LOG_HISTORY" ("table"), "\n" ("string"), "Where year(BREAKDOWN_DATE) ='%s' and month(BREAKDOWN_DATE) = '%s' and\n BREAKDOWN_STK_HOLD_ID ='%d' and STATION_ID_CID_TRIGGER= '%s'" ("condition")) -> (w866:string)
          n186 = Concatenate Strings("Select BREAKDOWN_IN_TIME,BREAKDOWN_OUT_TIME,DATEDIFF(MINUTE,BREAKDOWN_IN_TIME,BREAKDOWN_OUT_TIME)\nfrom STATION_3_LOG_HISTORY\n" ("string"), "Where year(BREAKDOWN_DATE) ='%s' and month(BREAKDOWN_DATE) = '%s' and\n BREAKDOWN_STK_HOLD_ID ='%d' and STATION_ID_CID_TRIGGER= '%s'" ("condition")) -> (w860:string)
          n187 = for {
            tunnel: w867 -> [w890]
            tunnel: w866 -> [w889]
            tunnel: w864 -> [w887] mode=indexing
            tunnel: w863 -> [w886]
            tunnel: [w885] -> w862
            tunnel: w861 -> [w884]
            shift-right: [w882] -> w868
            shift-left: string[][] [] ("Output Array") -> [w888]
            tunnel: w860 -> [w880]
            tunnel: [w879] -> w857
            shift-right: [w875] -> w858
            shift-left: string[][] [] ("Output Array") -> [w876]
            tunnel: [w874] -> w854
            tunnel: w855 -> [w873]
            tunnel: "3" -> [w872]
            n188 = for {
              tunnel: w889 -> [w912]
              tunnel: w890 -> [w902]
              tunnel: w887 -> [w901]
              tunnel: [w911] -> _ mode=indexing
              tunnel: w886 -> [w899]
              tunnel: [w909] -> w885
              tunnel: w884 -> [w900] mode=indexing
              shift-right: [w910] -> w883
              shift-left: w888 -> [w910]
              tunnel: [w905] -> w881 mode=indexing
              tunnel: w880 -> [w903]
              tunnel: [w896] -> w879
              tunnel: [w895] -> w878 mode=indexing
              shift-right: [w894] -> w877
              shift-left: w876 -> [w894]
              tunnel: [w892] -> w874
              tunnel: w873 -> [w892]
              tunnel: w872 -> [w891]
              n189 = Format Into String(format string=w903, w902, w901, w900, w891) -> (resulting string=w904:string)  [unwired: 2 in, 1 out]
              n190 = Format Into String(format string=w912, w902, w901, w900, w891) -> (resulting string=w911:string)  [unwired: 2 in, 1 out]
              n191 = call "Execute query.vi"("String"=w911, "connection reference"=w899) -> ("Table"=w908:string[][], "connection reference 2"=w909:T1)  [unwired: 6 in, 2 out]
              n192 = call "Execute query.vi"("String"=w904, "connection reference"=w899) -> ("Table"=w898:string[][], "connection reference 2"=w896:T1)  [unwired: 6 in, 2 out]
              n193 = Index Array(array=w908, index (row)=0 ("disabled index (col)")) -> (element=w906:string[])  [unwired: 1 in]
              n194 = Index Array(array=w898, index (col)=2 ("disabled index (col)")) -> (element=w897:string[])  [unwired: 1 in]
              n195 = Index Array(array=w897) -> (element=w895:string)  [unwired: 1 in]
              n196 = Index Array(array=w906) -> (element=w905:string)  [unwired: 1 in]
            }
            n197 = Build Array (concatenate)(w883, w881) -> (w882:string[][])
            n198 = Build Array (concatenate)(w877, w878) -> (w875:string[][])
          }
        }
        frame "1" {
          n199 = Array Size(array=w928) -> (size(s)=w927:i32)
          n200 = Concatenate Strings("select count(BREAKDOWN_STK_HOLD_ID) from " ("string"), "STATION_3_LOG_HISTORY" ("table"), "\n" ("string"), "Where year(BREAKDOWN_DATE) ='%s' and month(BREAKDOWN_DATE) = '%s' and\n BREAKDOWN_STK_HOLD_ID ='%d' and STATION_ID_CID_TRIGGER= '%s'and\nSHIFT_ID='%s'" ("condition")) -> (w930:string)
          n201 = Concatenate Strings("Select BREAKDOWN_IN_TIME,BREAKDOWN_OUT_TIME,DATEDIFF(MINUTE,BREAKDOWN_IN_TIME,BREAKDOWN_OUT_TIME)\nfrom STATION_3_LOG_HISTORY\n\n" ("string"), "Where year(BREAKDOWN_DATE) ='%s' and month(BREAKDOWN_DATE) = '%s' and\n BREAKDOWN_STK_HOLD_ID ='%d' and STATION_ID_CID_TRIGGER= '%s'and\nSHIFT_ID='%s'" ("condition")) -> (w920:string)
          n202 = for {
            tunnel: w931 -> [w956]
            tunnel: w930 -> [w955]
            tunnel: w928 -> [w953] mode=indexing
            tunnel: w927 -> [w952]
            tunnel: w926 -> [w951]
            tunnel: [w950] -> w925
            tunnel: w924 -> [w949]
            shift-right: [w947] -> w932
            shift-left: string[][] [] ("Output Array") -> [w954]
            tunnel: w920 -> [w945]
            shift-right: [w941] -> w922
            shift-left: string[][] [] ("Output Array") -> [w943]
            tunnel: [w940] -> w921
            tunnel: "3" -> [w939]
            tunnel: w916 -> [w938]
            tunnel: [w937] -> w914
            tunnel: w913 -> [w936]
            n203 = for {
              tunnel: w955 -> [w979]
              tunnel: w956 -> [w967]
              tunnel: w953 -> [w966]
              tunnel: [w978] -> _ mode=indexing
              tunnel: w952 -> [_]
              tunnel: w951 -> [w962]
              tunnel: [w976] -> w950
              tunnel: w949 -> [w965] mode=indexing
              shift-right: [w977] -> w948
              shift-left: w954 -> [w977]
              tunnel: [w973] -> w946 mode=indexing
              tunnel: w945 -> [w968]
              tunnel: [w964] -> w944 mode=indexing
              shift-right: [w963] -> w942
              shift-left: w943 -> [w963]
              tunnel: [w961] -> w940
              tunnel: w939 -> [w959]
              tunnel: w938 -> [w958]
              tunnel: [w957] -> w937
              tunnel: w936 -> [w957]
              n204 = Format Into String(format string=w979, w967, w966, w965, w959, w958) -> (resulting string=w978:string)  [unwired: 2 in, 1 out]
              n205 = Format Into String(format string=w968, w967, w966, w965, w959, w958) -> (resulting string=w971:string)  [unwired: 2 in, 1 out]
              n206 = call "Execute query.vi"("String"=w978, "connection reference"=w962) -> ("Table"=w972:string[][], "connection reference 2"=w976:T1)  [unwired: 6 in, 2 out]
              n207 = call "Execute query.vi"("String"=w971, "connection reference"=w962) -> ("Table"=w969:string[][], "connection reference 2"=w961:T1)  [unwired: 6 in, 2 out]
              n208 = Index Array(array=w972, index (row)=0 ("disabled index (col)")) -> (element=w974:string[])  [unwired: 1 in]
              n209 = Index Array(array=w969, index (col)=2 ("disabled index (col)")) -> (element=w970:string[])  [unwired: 1 in]
              n210 = Index Array(array=w970) -> (element=w964:string)  [unwired: 1 in]
              n211 = Index Array(array=w974) -> (element=w973:string)  [unwired: 1 in]
            }
            n212 = Build Array (concatenate)(w948, w946) -> (w947:string[][])
            n213 = Build Array (concatenate)(w942, w944) -> (w941:string[][])
          }
        }
        frame "2" {
          n214 = Array Size(array=w995) -> (size(s)=w994:i32)
          n215 = Concatenate Strings("select count(BREAKDOWN_STK_HOLD_ID) from " ("string"), "STATION_3_LOG_HISTORY" ("table"), "\n" ("string"), "Where year(BREAKDOWN_DATE) ='%s' and month(BREAKDOWN_DATE) = '%s' and\n BREAKDOWN_STK_HOLD_ID ='%d' and STATION_ID_CID_TRIGGER= '%s'and\nSHIFT_ID='%s'" ("condition")) -> (w997:string)
          n216 = Concatenate Strings("Select BREAKDOWN_IN_TIME,BREAKDOWN_OUT_TIME,DATEDIFF(MINUTE,BREAKDOWN_IN_TIME,BREAKDOWN_OUT_TIME)\nfrom STATION_3_LOG_HISTORY\n\n" ("string"), "Where year(BREAKDOWN_DATE) ='%s' and month(BREAKDOWN_DATE) = '%s' and\n BREAKDOWN_STK_HOLD_ID ='%d' and STATION_ID_CID_TRIGGER= '%s'and\nSHIFT_ID='%s'" ("condition")) -> (w987:string)
          n217 = for {
            tunnel: w998 -> [w1023]
            tunnel: w997 -> [w1022]
            tunnel: w995 -> [w1020] mode=indexing
            tunnel: w994 -> [w1019]
            tunnel: w993 -> [w1018]
            tunnel: [w1017] -> w992
            tunnel: w991 -> [w1016]
            shift-right: [w1014] -> w999
            shift-left: string[][] [] ("Output Array") -> [w1021]
            tunnel: w987 -> [w1012]
            shift-right: [w1008] -> w989
            shift-left: string[][] [] ("Output Array") -> [w1010]
            tunnel: [w1007] -> w988
            tunnel: "3" -> [w1006]
            tunnel: w983 -> [w1005]
            tunnel: [w1004] -> w981
            tunnel: w980 -> [w1003]
            n218 = for {
              tunnel: w1022 -> [w1046]
              tunnel: w1023 -> [w1034]
              tunnel: w1020 -> [w1033]
              tunnel: [w1045] -> _ mode=indexing
              tunnel: w1019 -> [_]
              tunnel: w1018 -> [w1029]
              tunnel: [w1043] -> w1017
              tunnel: w1016 -> [w1032] mode=indexing
              shift-right: [w1044] -> w1015
              shift-left: w1021 -> [w1044]
              tunnel: [w1040] -> w1013 mode=indexing
              tunnel: w1012 -> [w1035]
              tunnel: [w1031] -> w1011 mode=indexing
              shift-right: [w1030] -> w1009
              shift-left: w1010 -> [w1030]
              tunnel: [w1028] -> w1007
              tunnel: w1006 -> [w1026]
              tunnel: w1005 -> [w1025]
              tunnel: [w1024] -> w1004
              tunnel: w1003 -> [w1024]
              n219 = Format Into String(format string=w1046, w1034, w1033, w1032, w1026, w1025) -> (resulting string=w1045:string)  [unwired: 2 in, 1 out]
              n220 = Format Into String(format string=w1035, w1034, w1033, w1032, w1026, w1025) -> (resulting string=w1038:string)  [unwired: 2 in, 1 out]
              n221 = call "Execute query.vi"("String"=w1045, "connection reference"=w1029) -> ("Table"=w1039:string[][], "connection reference 2"=w1043:T1)  [unwired: 6 in, 2 out]
              n222 = call "Execute query.vi"("String"=w1038, "connection reference"=w1029) -> ("Table"=w1036:string[][], "connection reference 2"=w1028:T1)  [unwired: 6 in, 2 out]
              n223 = Index Array(array=w1039, index (row)=0 ("disabled index (col)")) -> (element=w1041:string[])  [unwired: 1 in]
              n224 = Index Array(array=w1036, index (col)=2 ("disabled index (col)")) -> (element=w1037:string[])  [unwired: 1 in]
              n225 = Index Array(array=w1037) -> (element=w1031:string)  [unwired: 1 in]
              n226 = Index Array(array=w1041) -> (element=w1040:string)  [unwired: 1 in]
            }
            n227 = Build Array (concatenate)(w1015, w1013) -> (w1014:string[][])
            n228 = Build Array (concatenate)(w1009, w1011) -> (w1008:string[][])
          }
        }
        frame "3" {
          n229 = Array Size(array=w1062) -> (size(s)=w1061:i32)
          n230 = Concatenate Strings("select count(BREAKDOWN_STK_HOLD_ID) from " ("string"), "STATION_3_LOG_HISTORY" ("table"), "\n" ("string"), "Where year(BREAKDOWN_DATE) ='%s' and month(BREAKDOWN_DATE) = '%s' and\n BREAKDOWN_STK_HOLD_ID ='%d' and STATION_ID_CID_TRIGGER= '%s'and\nSHIFT_ID='%s'" ("condition")) -> (w1064:string)
          n231 = Concatenate Strings("Select BREAKDOWN_IN_TIME,BREAKDOWN_OUT_TIME,DATEDIFF(MINUTE,BREAKDOWN_IN_TIME,BREAKDOWN_OUT_TIME)\nfrom STATION_3_LOG_HISTORY\n\n" ("string"), "Where year(BREAKDOWN_DATE) ='%s' and month(BREAKDOWN_DATE) = '%s' and\n BREAKDOWN_STK_HOLD_ID ='%d' and STATION_ID_CID_TRIGGER= '%s'and\nSHIFT_ID='%s'" ("condition")) -> (w1054:string)
          n232 = for {
            tunnel: w1065 -> [w1090]
            tunnel: w1064 -> [w1089]
            tunnel: w1062 -> [w1087] mode=indexing
            tunnel: w1061 -> [w1086]
            tunnel: w1060 -> [w1085]
            tunnel: [w1084] -> w1059
            tunnel: w1058 -> [w1083]
            shift-right: [w1081] -> w1066
            shift-left: string[][] [] ("Output Array") -> [w1088]
            tunnel: w1054 -> [w1079]
            shift-right: [w1075] -> w1056
            shift-left: string[][] [] ("Output Array") -> [w1077]
            tunnel: [w1074] -> w1055
            tunnel: "3" -> [w1073]
            tunnel: w1050 -> [w1072]
            tunnel: [w1071] -> w1048
            tunnel: w1047 -> [w1070]
            n233 = for {
              tunnel: w1089 -> [w1113]
              tunnel: w1090 -> [w1101]
              tunnel: w1087 -> [w1100]
              tunnel: [w1112] -> _ mode=indexing
              tunnel: w1086 -> [_]
              tunnel: w1085 -> [w1096]
              tunnel: [w1110] -> w1084
              tunnel: w1083 -> [w1099] mode=indexing
              shift-right: [w1111] -> w1082
              shift-left: w1088 -> [w1111]
              tunnel: [w1107] -> w1080 mode=indexing
              tunnel: w1079 -> [w1102]
              tunnel: [w1098] -> w1078 mode=indexing
              shift-right: [w1097] -> w1076
              shift-left: w1077 -> [w1097]
              tunnel: [w1095] -> w1074
              tunnel: w1073 -> [w1093]
              tunnel: w1072 -> [w1092]
              tunnel: [w1091] -> w1071
              tunnel: w1070 -> [w1091]
              n234 = Format Into String(format string=w1113, w1101, w1100, w1099, w1093, w1092) -> (resulting string=w1112:string)  [unwired: 2 in, 1 out]
              n235 = Format Into String(format string=w1102, w1101, w1100, w1099, w1093, w1092) -> (resulting string=w1105:string)  [unwired: 2 in, 1 out]
              n236 = call "Execute query.vi"("String"=w1112, "connection reference"=w1096) -> ("Table"=w1106:string[][], "connection reference 2"=w1110:T1)  [unwired: 6 in, 2 out]
              n237 = call "Execute query.vi"("String"=w1105, "connection reference"=w1096) -> ("Table"=w1103:string[][], "connection reference 2"=w1095:T1)  [unwired: 6 in, 2 out]
              n238 = Index Array(array=w1106, index (row)=0 ("disabled index (col)")) -> (element=w1108:string[])  [unwired: 1 in]
              n239 = Index Array(array=w1103, index (col)=2 ("disabled index (col)")) -> (element=w1104:string[])  [unwired: 1 in]
              n240 = Index Array(array=w1104) -> (element=w1098:string)  [unwired: 1 in]
              n241 = Index Array(array=w1108) -> (element=w1107:string)  [unwired: 1 in]
            }
            n242 = Build Array (concatenate)(w1082, w1080) -> (w1081:string[][])
            n243 = Build Array (concatenate)(w1076, w1078) -> (w1075:string[][])
          }
        }
      }
    }
    frame "ST 4" {
      n244 = case shown="\"ALL\"" w1125 {
        selector: w1125 -> [_ _ w1193 w1260 w1327]
        tunnel: w1124 -> [_ _ _ _ _]
        tunnel: w1123 -> [_ w1144 w1208 w1275 w1342]
        tunnel: w1122 -> [_ w1141 w1205 w1272 w1339]
        tunnel: [_ w1145 w1209 w1276 w1343] -> w1121
        tunnel: w1120 -> [w1127 w1140 w1203 w1270 w1337]
        tunnel: [w1127 w1139 w1202 w1269 w1336] -> w1119
        tunnel: w1118 -> [_ w1138 w1201 w1268 w1335]
        tunnel: [_ w1135 w1199 w1266 w1333] -> w1117
        tunnel: [_ w1134 w1198 w1265 w1332] -> w1116
        tunnel: w1115 -> [w1126 w1132 w1190 w1257 w1324]
        tunnel: [w1126 w1131 w1191 w1258 w1325] -> w1114
        frame "False", Default {
        }
        frame "ALL" {
          n245 = Concatenate Strings("select count(BREAKDOWN_STK_HOLD_ID) from " ("string"), "STATION_4_LOG_HISTORY" ("table"), "\n" ("string"), "Where year(BREAKDOWN_DATE) ='%s' and month(BREAKDOWN_DATE) = '%s' and\n BREAKDOWN_STK_HOLD_ID ='%d' and STATION_ID_CID_TRIGGER= '%s'" ("condition")) -> (w1143:string)
          n246 = Concatenate Strings("Select BREAKDOWN_IN_TIME,BREAKDOWN_OUT_TIME,DATEDIFF(MINUTE,BREAKDOWN_IN_TIME,BREAKDOWN_OUT_TIME)\nfrom STATION_4_LOG_HISTORY\n" ("string"), "Where year(BREAKDOWN_DATE) ='%s' and month(BREAKDOWN_DATE) = '%s' and\n BREAKDOWN_STK_HOLD_ID ='%d' and STATION_ID_CID_TRIGGER= '%s'" ("condition")) -> (w1137:string)
          n247 = for {
            tunnel: w1144 -> [w1167]
            tunnel: w1143 -> [w1166]
            tunnel: w1141 -> [w1164] mode=indexing
            tunnel: w1140 -> [w1163]
            tunnel: [w1162] -> w1139
            tunnel: w1138 -> [w1161]
            shift-right: [w1159] -> w1145
            shift-left: string[][] [] ("Output Array") -> [w1165]
            tunnel: w1137 -> [w1157]
            tunnel: [w1156] -> w1134
            shift-right: [w1152] -> w1135
            shift-left: string[][] [] ("Output Array") -> [w1153]
            tunnel: [w1151] -> w1131
            tunnel: w1132 -> [w1150]
            tunnel: "4" -> [w1149]
            n248 = for {
              tunnel: w1166 -> [w1189]
              tunnel: w1167 -> [w1179]
              tunnel: w1164 -> [w1178]
              tunnel: [w1188] -> _ mode=indexing
              tunnel: w1163 -> [w1176]
              tunnel: [w1186] -> w1162
              tunnel: w1161 -> [w1177] mode=indexing
              shift-right: [w1187] -> w1160
              shift-left: w1165 -> [w1187]
              tunnel: [w1182] -> w1158 mode=indexing
              tunnel: w1157 -> [w1180]
              tunnel: [w1173] -> w1156
              tunnel: [w1172] -> w1155 mode=indexing
              shift-right: [w1171] -> w1154
              shift-left: w1153 -> [w1171]
              tunnel: [w1169] -> w1151
              tunnel: w1150 -> [w1169]
              tunnel: w1149 -> [w1168]
              n249 = Format Into String(format string=w1180, w1179, w1178, w1177, w1168) -> (resulting string=w1181:string)  [unwired: 2 in, 1 out]
              n250 = Format Into String(format string=w1189, w1179, w1178, w1177, w1168) -> (resulting string=w1188:string)  [unwired: 2 in, 1 out]
              n251 = call "Execute query.vi"("String"=w1188, "connection reference"=w1176) -> ("Table"=w1185:string[][], "connection reference 2"=w1186:T1)  [unwired: 6 in, 2 out]
              n252 = call "Execute query.vi"("String"=w1181, "connection reference"=w1176) -> ("Table"=w1175:string[][], "connection reference 2"=w1173:T1)  [unwired: 6 in, 2 out]
              n253 = Index Array(array=w1185, index (row)=0 ("disabled index (col)")) -> (element=w1183:string[])  [unwired: 1 in]
              n254 = Index Array(array=w1175, index (col)=2 ("disabled index (col)")) -> (element=w1174:string[])  [unwired: 1 in]
              n255 = Index Array(array=w1174) -> (element=w1172:string)  [unwired: 1 in]
              n256 = Index Array(array=w1183) -> (element=w1182:string)  [unwired: 1 in]
            }
            n257 = Build Array (concatenate)(w1160, w1158) -> (w1159:string[][])
            n258 = Build Array (concatenate)(w1154, w1155) -> (w1152:string[][])
          }
        }
        frame "1" {
          n259 = Array Size(array=w1205) -> (size(s)=w1204:i32)
          n260 = Concatenate Strings("select count(BREAKDOWN_STK_HOLD_ID) from " ("string"), "STATION_4_LOG_HISTORY" ("table"), "\n" ("string"), "Where year(BREAKDOWN_DATE) ='%s' and month(BREAKDOWN_DATE) = '%s' and\n BREAKDOWN_STK_HOLD_ID ='%d' and STATION_ID_CID_TRIGGER= '%s'and\nSHIFT_ID='%s'" ("condition")) -> (w1207:string)
          n261 = Concatenate Strings("Select BREAKDOWN_IN_TIME,BREAKDOWN_OUT_TIME,DATEDIFF(MINUTE,BREAKDOWN_IN_TIME,BREAKDOWN_OUT_TIME)\nfrom STATION_4_LOG_HISTORY\n\n" ("string"), "Where year(BREAKDOWN_DATE) ='%s' and month(BREAKDOWN_DATE) = '%s' and\n BREAKDOWN_STK_HOLD_ID ='%d' and STATION_ID_CID_TRIGGER= '%s'and\nSHIFT_ID='%s'" ("condition")) -> (w1197:string)
          n262 = for {
            tunnel: w1208 -> [w1233]
            tunnel: w1207 -> [w1232]
            tunnel: w1205 -> [w1230] mode=indexing
            tunnel: w1204 -> [w1229]
            tunnel: w1203 -> [w1228]
            tunnel: [w1227] -> w1202
            tunnel: w1201 -> [w1226]
            shift-right: [w1224] -> w1209
            shift-left: string[][] [] ("Output Array") -> [w1231]
            tunnel: w1197 -> [w1222]
            shift-right: [w1218] -> w1199
            shift-left: string[][] [] ("Output Array") -> [w1220]
            tunnel: [w1217] -> w1198
            tunnel: "4" -> [w1216]
            tunnel: w1193 -> [w1215]
            tunnel: [w1214] -> w1191
            tunnel: w1190 -> [w1213]
            n263 = for {
              tunnel: w1232 -> [w1256]
              tunnel: w1233 -> [w1244]
              tunnel: w1230 -> [w1243]
              tunnel: [w1255] -> _ mode=indexing
              tunnel: w1229 -> [_]
              tunnel: w1228 -> [w1239]
              tunnel: [w1253] -> w1227
              tunnel: w1226 -> [w1242] mode=indexing
              shift-right: [w1254] -> w1225
              shift-left: w1231 -> [w1254]
              tunnel: [w1250] -> w1223 mode=indexing
              tunnel: w1222 -> [w1245]
              tunnel: [w1241] -> w1221 mode=indexing
              shift-right: [w1240] -> w1219
              shift-left: w1220 -> [w1240]
              tunnel: [w1238] -> w1217
              tunnel: w1216 -> [w1236]
              tunnel: w1215 -> [w1235]
              tunnel: [w1234] -> w1214
              tunnel: w1213 -> [w1234]
              n264 = Format Into String(format string=w1256, w1244, w1243, w1242, w1236, w1235) -> (resulting string=w1255:string)  [unwired: 2 in, 1 out]
              n265 = Format Into String(format string=w1245, w1244, w1243, w1242, w1236, w1235) -> (resulting string=w1248:string)  [unwired: 2 in, 1 out]
              n266 = call "Execute query.vi"("String"=w1255, "connection reference"=w1239) -> ("Table"=w1249:string[][], "connection reference 2"=w1253:T1)  [unwired: 6 in, 2 out]
              n267 = call "Execute query.vi"("String"=w1248, "connection reference"=w1239) -> ("Table"=w1246:string[][], "connection reference 2"=w1238:T1)  [unwired: 6 in, 2 out]
              n268 = Index Array(array=w1249, index (row)=0 ("disabled index (col)")) -> (element=w1251:string[])  [unwired: 1 in]
              n269 = Index Array(array=w1246, index (col)=2 ("disabled index (col)")) -> (element=w1247:string[])  [unwired: 1 in]
              n270 = Index Array(array=w1247) -> (element=w1241:string)  [unwired: 1 in]
              n271 = Index Array(array=w1251) -> (element=w1250:string)  [unwired: 1 in]
            }
            n272 = Build Array (concatenate)(w1225, w1223) -> (w1224:string[][])
            n273 = Build Array (concatenate)(w1219, w1221) -> (w1218:string[][])
          }
        }
        frame "2" {
          n274 = Array Size(array=w1272) -> (size(s)=w1271:i32)
          n275 = Concatenate Strings("select count(BREAKDOWN_STK_HOLD_ID) from " ("string"), "STATION_4_LOG_HISTORY" ("table"), "\n" ("string"), "Where year(BREAKDOWN_DATE) ='%s' and month(BREAKDOWN_DATE) = '%s' and\n BREAKDOWN_STK_HOLD_ID ='%d' and STATION_ID_CID_TRIGGER= '%s'and\nSHIFT_ID='%s'" ("condition")) -> (w1274:string)
          n276 = Concatenate Strings("Select BREAKDOWN_IN_TIME,BREAKDOWN_OUT_TIME,DATEDIFF(MINUTE,BREAKDOWN_IN_TIME,BREAKDOWN_OUT_TIME)\nfrom STATION_4_LOG_HISTORY\n\n" ("string"), "Where year(BREAKDOWN_DATE) ='%s' and month(BREAKDOWN_DATE) = '%s' and\n BREAKDOWN_STK_HOLD_ID ='%d' and STATION_ID_CID_TRIGGER= '%s'and\nSHIFT_ID='%s'" ("condition")) -> (w1264:string)
          n277 = for {
            tunnel: w1275 -> [w1300]
            tunnel: w1274 -> [w1299]
            tunnel: w1272 -> [w1297] mode=indexing
            tunnel: w1271 -> [w1296]
            tunnel: w1270 -> [w1295]
            tunnel: [w1294] -> w1269
            tunnel: w1268 -> [w1293]
            shift-right: [w1291] -> w1276
            shift-left: string[][] [] ("Output Array") -> [w1298]
            tunnel: w1264 -> [w1289]
            shift-right: [w1285] -> w1266
            shift-left: string[][] [] ("Output Array") -> [w1287]
            tunnel: [w1284] -> w1265
            tunnel: "4" -> [w1283]
            tunnel: w1260 -> [w1282]
            tunnel: [w1281] -> w1258
            tunnel: w1257 -> [w1280]
            n278 = for {
              tunnel: w1299 -> [w1323]
              tunnel: w1300 -> [w1311]
              tunnel: w1297 -> [w1310]
              tunnel: [w1322] -> _ mode=indexing
              tunnel: w1296 -> [_]
              tunnel: w1295 -> [w1306]
              tunnel: [w1320] -> w1294
              tunnel: w1293 -> [w1309] mode=indexing
              shift-right: [w1321] -> w1292
              shift-left: w1298 -> [w1321]
              tunnel: [w1317] -> w1290 mode=indexing
              tunnel: w1289 -> [w1312]
              tunnel: [w1308] -> w1288 mode=indexing
              shift-right: [w1307] -> w1286
              shift-left: w1287 -> [w1307]
              tunnel: [w1305] -> w1284
              tunnel: w1283 -> [w1303]
              tunnel: w1282 -> [w1302]
              tunnel: [w1301] -> w1281
              tunnel: w1280 -> [w1301]
              n279 = Format Into String(format string=w1323, w1311, w1310, w1309, w1303, w1302) -> (resulting string=w1322:string)  [unwired: 2 in, 1 out]
              n280 = Format Into String(format string=w1312, w1311, w1310, w1309, w1303, w1302) -> (resulting string=w1315:string)  [unwired: 2 in, 1 out]
              n281 = call "Execute query.vi"("String"=w1322, "connection reference"=w1306) -> ("Table"=w1316:string[][], "connection reference 2"=w1320:T1)  [unwired: 6 in, 2 out]
              n282 = call "Execute query.vi"("String"=w1315, "connection reference"=w1306) -> ("Table"=w1313:string[][], "connection reference 2"=w1305:T1)  [unwired: 6 in, 2 out]
              n283 = Index Array(array=w1316, index (row)=0 ("disabled index (col)")) -> (element=w1318:string[])  [unwired: 1 in]
              n284 = Index Array(array=w1313, index (col)=2 ("disabled index (col)")) -> (element=w1314:string[])  [unwired: 1 in]
              n285 = Index Array(array=w1314) -> (element=w1308:string)  [unwired: 1 in]
              n286 = Index Array(array=w1318) -> (element=w1317:string)  [unwired: 1 in]
            }
            n287 = Build Array (concatenate)(w1292, w1290) -> (w1291:string[][])
            n288 = Build Array (concatenate)(w1286, w1288) -> (w1285:string[][])
          }
        }
        frame "3" {
          n289 = Array Size(array=w1339) -> (size(s)=w1338:i32)
          n290 = Concatenate Strings("select count(BREAKDOWN_STK_HOLD_ID) from " ("string"), "STATION_4_LOG_HISTORY" ("table"), "\n" ("string"), "Where year(BREAKDOWN_DATE) ='%s' and month(BREAKDOWN_DATE) = '%s' and\n BREAKDOWN_STK_HOLD_ID ='%d' and STATION_ID_CID_TRIGGER= '%s'and\nSHIFT_ID='%s'" ("condition")) -> (w1341:string)
          n291 = Concatenate Strings("Select BREAKDOWN_IN_TIME,BREAKDOWN_OUT_TIME,DATEDIFF(MINUTE,BREAKDOWN_IN_TIME,BREAKDOWN_OUT_TIME)\nfrom STATION_4_LOG_HISTORY\n\n" ("string"), "Where year(BREAKDOWN_DATE) ='%s' and month(BREAKDOWN_DATE) = '%s' and\n BREAKDOWN_STK_HOLD_ID ='%d' and STATION_ID_CID_TRIGGER= '%s'and\nSHIFT_ID='%s'" ("condition")) -> (w1331:string)
          n292 = for {
            tunnel: w1342 -> [w1367]
            tunnel: w1341 -> [w1366]
            tunnel: w1339 -> [w1364] mode=indexing
            tunnel: w1338 -> [w1363]
            tunnel: w1337 -> [w1362]
            tunnel: [w1361] -> w1336
            tunnel: w1335 -> [w1360]
            shift-right: [w1358] -> w1343
            shift-left: string[][] [] ("Output Array") -> [w1365]
            tunnel: w1331 -> [w1356]
            shift-right: [w1352] -> w1333
            shift-left: string[][] [] ("Output Array") -> [w1354]
            tunnel: [w1351] -> w1332
            tunnel: "4" -> [w1350]
            tunnel: w1327 -> [w1349]
            tunnel: [w1348] -> w1325
            tunnel: w1324 -> [w1347]
            n293 = for {
              tunnel: w1366 -> [w1390]
              tunnel: w1367 -> [w1378]
              tunnel: w1364 -> [w1377]
              tunnel: [w1389] -> _ mode=indexing
              tunnel: w1363 -> [_]
              tunnel: w1362 -> [w1373]
              tunnel: [w1387] -> w1361
              tunnel: w1360 -> [w1376] mode=indexing
              shift-right: [w1388] -> w1359
              shift-left: w1365 -> [w1388]
              tunnel: [w1384] -> w1357 mode=indexing
              tunnel: w1356 -> [w1379]
              tunnel: [w1375] -> w1355 mode=indexing
              shift-right: [w1374] -> w1353
              shift-left: w1354 -> [w1374]
              tunnel: [w1372] -> w1351
              tunnel: w1350 -> [w1370]
              tunnel: w1349 -> [w1369]
              tunnel: [w1368] -> w1348
              tunnel: w1347 -> [w1368]
              n294 = Format Into String(format string=w1390, w1378, w1377, w1376, w1370, w1369) -> (resulting string=w1389:string)  [unwired: 2 in, 1 out]
              n295 = Format Into String(format string=w1379, w1378, w1377, w1376, w1370, w1369) -> (resulting string=w1382:string)  [unwired: 2 in, 1 out]
              n296 = call "Execute query.vi"("String"=w1389, "connection reference"=w1373) -> ("Table"=w1383:string[][], "connection reference 2"=w1387:T1)  [unwired: 6 in, 2 out]
              n297 = call "Execute query.vi"("String"=w1382, "connection reference"=w1373) -> ("Table"=w1380:string[][], "connection reference 2"=w1372:T1)  [unwired: 6 in, 2 out]
              n298 = Index Array(array=w1383, index (row)=0 ("disabled index (col)")) -> (element=w1385:string[])  [unwired: 1 in]
              n299 = Index Array(array=w1380, index (col)=2 ("disabled index (col)")) -> (element=w1381:string[])  [unwired: 1 in]
              n300 = Index Array(array=w1381) -> (element=w1375:string)  [unwired: 1 in]
              n301 = Index Array(array=w1385) -> (element=w1384:string)  [unwired: 1 in]
            }
            n302 = Build Array (concatenate)(w1359, w1357) -> (w1358:string[][])
            n303 = Build Array (concatenate)(w1353, w1355) -> (w1352:string[][])
          }
        }
      }
    }
    frame "ST 5" {
      n304 = case shown="\"2\"" w1402 {
        selector: w1402 -> [_ _ w1470 w1537 w1604]
        tunnel: w1401 -> [_ _ _ _ _]
        tunnel: w1400 -> [_ w1421 w1485 w1552 w1619]
        tunnel: w1399 -> [_ w1418 w1482 w1549 w1616]
        tunnel: [_ w1422 w1486 w1553 w1620] -> w1398
        tunnel: w1397 -> [w1404 w1417 w1480 w1547 w1614]
        tunnel: [w1404 w1416 w1479 w1546 w1613] -> w1396
        tunnel: w1395 -> [_ w1415 w1478 w1545 w1612]
        tunnel: [_ w1412 w1476 w1543 w1610] -> w1394
        tunnel: [_ w1411 w1475 w1542 w1609] -> w1393
        tunnel: w1392 -> [w1403 w1409 w1467 w1534 w1601]
        tunnel: [w1403 w1408 w1468 w1535 w1602] -> w1391
        frame "False", Default {
        }
        frame "ALL" {
          n305 = Concatenate Strings("select count(BREAKDOWN_STK_HOLD_ID) from " ("string"), "STATION_5_LOG_HISTORY" ("table"), "\n" ("string"), "Where year(BREAKDOWN_DATE) ='%s' and month(BREAKDOWN_DATE) = '%s' and\n BREAKDOWN_STK_HOLD_ID ='%d' and STATION_ID_CID_TRIGGER= '%s'" ("condition")) -> (w1420:string)
          n306 = Concatenate Strings("Select BREAKDOWN_IN_TIME,BREAKDOWN_OUT_TIME,DATEDIFF(MINUTE,BREAKDOWN_IN_TIME,BREAKDOWN_OUT_TIME)\nfrom STATION_5_LOG_HISTORY\n" ("string"), "Where year(BREAKDOWN_DATE) ='%s' and month(BREAKDOWN_DATE) = '%s' and\n BREAKDOWN_STK_HOLD_ID ='%d' and STATION_ID_CID_TRIGGER= '%s'" ("condition")) -> (w1414:string)
          n307 = for {
            tunnel: w1421 -> [w1444]
            tunnel: w1420 -> [w1443]
            tunnel: w1418 -> [w1441] mode=indexing
            tunnel: w1417 -> [w1440]
            tunnel: [w1439] -> w1416
            tunnel: w1415 -> [w1438]
            shift-right: [w1436] -> w1422
            shift-left: string[][] [] ("Output Array") -> [w1442]
            tunnel: w1414 -> [w1434]
            tunnel: [w1433] -> w1411
            shift-right: [w1429] -> w1412
            shift-left: string[][] [] ("Output Array") -> [w1430]
            tunnel: [w1428] -> w1408
            tunnel: w1409 -> [w1427]
            tunnel: "5" -> [w1426]
            n308 = for {
              tunnel: w1443 -> [w1466]
              tunnel: w1444 -> [w1456]
              tunnel: w1441 -> [w1455]
              tunnel: [w1465] -> _ mode=indexing
              tunnel: w1440 -> [w1453]
              tunnel: [w1463] -> w1439
              tunnel: w1438 -> [w1454] mode=indexing
              shift-right: [w1464] -> w1437
              shift-left: w1442 -> [w1464]
              tunnel: [w1459] -> w1435 mode=indexing
              tunnel: w1434 -> [w1457]
              tunnel: [w1450] -> w1433
              tunnel: [w1449] -> w1432 mode=indexing
              shift-right: [w1448] -> w1431
              shift-left: w1430 -> [w1448]
              tunnel: [w1446] -> w1428
              tunnel: w1427 -> [w1446]
              tunnel: w1426 -> [w1445]
              n309 = Format Into String(format string=w1457, w1456, w1455, w1454, w1445) -> (resulting string=w1458:string)  [unwired: 2 in, 1 out]
              n310 = Format Into String(format string=w1466, w1456, w1455, w1454, w1445) -> (resulting string=w1465:string)  [unwired: 2 in, 1 out]
              n311 = call "Execute query.vi"("String"=w1465, "connection reference"=w1453) -> ("Table"=w1462:string[][], "connection reference 2"=w1463:T1)  [unwired: 6 in, 2 out]
              n312 = call "Execute query.vi"("String"=w1458, "connection reference"=w1453) -> ("Table"=w1452:string[][], "connection reference 2"=w1450:T1)  [unwired: 6 in, 2 out]
              n313 = Index Array(array=w1462, index (row)=0 ("disabled index (col)")) -> (element=w1460:string[])  [unwired: 1 in]
              n314 = Index Array(array=w1452, index (col)=2 ("disabled index (col)")) -> (element=w1451:string[])  [unwired: 1 in]
              n315 = Index Array(array=w1451) -> (element=w1449:string)  [unwired: 1 in]
              n316 = Index Array(array=w1460) -> (element=w1459:string)  [unwired: 1 in]
            }
            n317 = Build Array (concatenate)(w1437, w1435) -> (w1436:string[][])
            n318 = Build Array (concatenate)(w1431, w1432) -> (w1429:string[][])
          }
        }
        frame "1" {
          n319 = Array Size(array=w1482) -> (size(s)=w1481:i32)
          n320 = Concatenate Strings("select count(BREAKDOWN_STK_HOLD_ID) from " ("string"), "STATION_5_LOG_HISTORY" ("table"), "\n" ("string"), "Where year(BREAKDOWN_DATE) ='%s' and month(BREAKDOWN_DATE) = '%s' and\n BREAKDOWN_STK_HOLD_ID ='%d' and STATION_ID_CID_TRIGGER= '%s'and\nSHIFT_ID='%s'" ("condition")) -> (w1484:string)
          n321 = Concatenate Strings("Select BREAKDOWN_IN_TIME,BREAKDOWN_OUT_TIME,DATEDIFF(MINUTE,BREAKDOWN_IN_TIME,BREAKDOWN_OUT_TIME)\nfrom STATION_5_LOG_HISTORY\n\n" ("string"), "Where year(BREAKDOWN_DATE) ='%s' and month(BREAKDOWN_DATE) = '%s' and\n BREAKDOWN_STK_HOLD_ID ='%d' and STATION_ID_CID_TRIGGER= '%s'and\nSHIFT_ID='%s'" ("condition")) -> (w1474:string)
          n322 = for {
            tunnel: w1485 -> [w1510]
            tunnel: w1484 -> [w1509]
            tunnel: w1482 -> [w1507] mode=indexing
            tunnel: w1481 -> [w1506]
            tunnel: w1480 -> [w1505]
            tunnel: [w1504] -> w1479
            tunnel: w1478 -> [w1503]
            shift-right: [w1501] -> w1486
            shift-left: string[][] [] ("Output Array") -> [w1508]
            tunnel: w1474 -> [w1499]
            shift-right: [w1495] -> w1476
            shift-left: string[][] [] ("Output Array") -> [w1497]
            tunnel: [w1494] -> w1475
            tunnel: "5" -> [w1493]
            tunnel: w1470 -> [w1492]
            tunnel: [w1491] -> w1468
            tunnel: w1467 -> [w1490]
            n323 = for {
              tunnel: w1509 -> [w1533]
              tunnel: w1510 -> [w1521]
              tunnel: w1507 -> [w1520]
              tunnel: [w1532] -> _ mode=indexing
              tunnel: w1506 -> [_]
              tunnel: w1505 -> [w1516]
              tunnel: [w1530] -> w1504
              tunnel: w1503 -> [w1519] mode=indexing
              shift-right: [w1531] -> w1502
              shift-left: w1508 -> [w1531]
              tunnel: [w1527] -> w1500 mode=indexing
              tunnel: w1499 -> [w1522]
              tunnel: [w1518] -> w1498 mode=indexing
              shift-right: [w1517] -> w1496
              shift-left: w1497 -> [w1517]
              tunnel: [w1515] -> w1494
              tunnel: w1493 -> [w1513]
              tunnel: w1492 -> [w1512]
              tunnel: [w1511] -> w1491
              tunnel: w1490 -> [w1511]
              n324 = Format Into String(format string=w1533, w1521, w1520, w1519, w1513, w1512) -> (resulting string=w1532:string)  [unwired: 2 in, 1 out]
              n325 = Format Into String(format string=w1522, w1521, w1520, w1519, w1513, w1512) -> (resulting string=w1525:string)  [unwired: 2 in, 1 out]
              n326 = call "Execute query.vi"("String"=w1532, "connection reference"=w1516) -> ("Table"=w1526:string[][], "connection reference 2"=w1530:T1)  [unwired: 6 in, 2 out]
              n327 = call "Execute query.vi"("String"=w1525, "connection reference"=w1516) -> ("Table"=w1523:string[][], "connection reference 2"=w1515:T1)  [unwired: 6 in, 2 out]
              n328 = Index Array(array=w1526, index (row)=0 ("disabled index (col)")) -> (element=w1528:string[])  [unwired: 1 in]
              n329 = Index Array(array=w1523, index (col)=2 ("disabled index (col)")) -> (element=w1524:string[])  [unwired: 1 in]
              n330 = Index Array(array=w1524) -> (element=w1518:string)  [unwired: 1 in]
              n331 = Index Array(array=w1528) -> (element=w1527:string)  [unwired: 1 in]
            }
            n332 = Build Array (concatenate)(w1502, w1500) -> (w1501:string[][])
            n333 = Build Array (concatenate)(w1496, w1498) -> (w1495:string[][])
          }
        }
        frame "2" {
          n334 = Array Size(array=w1549) -> (size(s)=w1548:i32)
          n335 = Concatenate Strings("select count(BREAKDOWN_STK_HOLD_ID) from " ("string"), "STATION_5_LOG_HISTORY" ("table"), "\n" ("string"), "Where year(BREAKDOWN_DATE) ='%s' and month(BREAKDOWN_DATE) = '%s' and\n BREAKDOWN_STK_HOLD_ID ='%d' and STATION_ID_CID_TRIGGER= '%s'and\nSHIFT_ID='%s'" ("condition")) -> (w1551:string)
          n336 = Concatenate Strings("Select BREAKDOWN_IN_TIME,BREAKDOWN_OUT_TIME,DATEDIFF(MINUTE,BREAKDOWN_IN_TIME,BREAKDOWN_OUT_TIME)\nfrom STATION_5_LOG_HISTORY\n\n" ("string"), "Where year(BREAKDOWN_DATE) ='%s' and month(BREAKDOWN_DATE) = '%s' and\n BREAKDOWN_STK_HOLD_ID ='%d' and STATION_ID_CID_TRIGGER= '%s'and\nSHIFT_ID='%s'" ("condition")) -> (w1541:string)
          n337 = for {
            tunnel: w1552 -> [w1577]
            tunnel: w1551 -> [w1576]
            tunnel: w1549 -> [w1574] mode=indexing
            tunnel: w1548 -> [w1573]
            tunnel: w1547 -> [w1572]
            tunnel: [w1571] -> w1546
            tunnel: w1545 -> [w1570]
            shift-right: [w1568] -> w1553
            shift-left: string[][] [] ("Output Array") -> [w1575]
            tunnel: w1541 -> [w1566]
            shift-right: [w1562] -> w1543
            shift-left: string[][] [] ("Output Array") -> [w1564]
            tunnel: [w1561] -> w1542
            tunnel: "5" -> [w1560]
            tunnel: w1537 -> [w1559]
            tunnel: [w1558] -> w1535
            tunnel: w1534 -> [w1557]
            n338 = for {
              tunnel: w1576 -> [w1600]
              tunnel: w1577 -> [w1588]
              tunnel: w1574 -> [w1587]
              tunnel: [w1599] -> _ mode=indexing
              tunnel: w1573 -> [_]
              tunnel: w1572 -> [w1583]
              tunnel: [w1597] -> w1571
              tunnel: w1570 -> [w1586] mode=indexing
              shift-right: [w1598] -> w1569
              shift-left: w1575 -> [w1598]
              tunnel: [w1594] -> w1567 mode=indexing
              tunnel: w1566 -> [w1589]
              tunnel: [w1585] -> w1565 mode=indexing
              shift-right: [w1584] -> w1563
              shift-left: w1564 -> [w1584]
              tunnel: [w1582] -> w1561
              tunnel: w1560 -> [w1580]
              tunnel: w1559 -> [w1579]
              tunnel: [w1578] -> w1558
              tunnel: w1557 -> [w1578]
              n339 = Format Into String(format string=w1600, w1588, w1587, w1586, w1580, w1579) -> (resulting string=w1599:string)  [unwired: 2 in, 1 out]
              n340 = Format Into String(format string=w1589, w1588, w1587, w1586, w1580, w1579) -> (resulting string=w1592:string)  [unwired: 2 in, 1 out]
              n341 = call "Execute query.vi"("String"=w1599, "connection reference"=w1583) -> ("Table"=w1593:string[][], "connection reference 2"=w1597:T1)  [unwired: 6 in, 2 out]
              n342 = call "Execute query.vi"("String"=w1592, "connection reference"=w1583) -> ("Table"=w1590:string[][], "connection reference 2"=w1582:T1)  [unwired: 6 in, 2 out]
              n343 = Index Array(array=w1593, index (row)=0 ("disabled index (col)")) -> (element=w1595:string[])  [unwired: 1 in]
              n344 = Index Array(array=w1590, index (col)=2 ("disabled index (col)")) -> (element=w1591:string[])  [unwired: 1 in]
              n345 = Index Array(array=w1591) -> (element=w1585:string)  [unwired: 1 in]
              n346 = Index Array(array=w1595) -> (element=w1594:string)  [unwired: 1 in]
            }
            n347 = Build Array (concatenate)(w1569, w1567) -> (w1568:string[][])
            n348 = Build Array (concatenate)(w1563, w1565) -> (w1562:string[][])
          }
        }
        frame "3" {
          n349 = Array Size(array=w1616) -> (size(s)=w1615:i32)
          n350 = Concatenate Strings("select count(BREAKDOWN_STK_HOLD_ID) from " ("string"), "STATION_5_LOG_HISTORY" ("table"), "\n" ("string"), "Where year(BREAKDOWN_DATE) ='%s' and month(BREAKDOWN_DATE) = '%s' and\n BREAKDOWN_STK_HOLD_ID ='%d' and STATION_ID_CID_TRIGGER= '%s'and\nSHIFT_ID='%s'" ("condition")) -> (w1618:string)
          n351 = Concatenate Strings("Select BREAKDOWN_IN_TIME,BREAKDOWN_OUT_TIME,DATEDIFF(MINUTE,BREAKDOWN_IN_TIME,BREAKDOWN_OUT_TIME)\nfrom STATION_5_LOG_HISTORY\n\n" ("string"), "Where year(BREAKDOWN_DATE) ='%s' and month(BREAKDOWN_DATE) = '%s' and\n BREAKDOWN_STK_HOLD_ID ='%d' and STATION_ID_CID_TRIGGER= '%s'and\nSHIFT_ID='%s'" ("condition")) -> (w1608:string)
          n352 = for {
            tunnel: w1619 -> [w1644]
            tunnel: w1618 -> [w1643]
            tunnel: w1616 -> [w1641] mode=indexing
            tunnel: w1615 -> [w1640]
            tunnel: w1614 -> [w1639]
            tunnel: [w1638] -> w1613
            tunnel: w1612 -> [w1637]
            shift-right: [w1635] -> w1620
            shift-left: string[][] [] ("Output Array") -> [w1642]
            tunnel: w1608 -> [w1633]
            shift-right: [w1629] -> w1610
            shift-left: string[][] [] ("Output Array") -> [w1631]
            tunnel: [w1628] -> w1609
            tunnel: "5" -> [w1627]
            tunnel: w1604 -> [w1626]
            tunnel: [w1625] -> w1602
            tunnel: w1601 -> [w1624]
            n353 = for {
              tunnel: w1643 -> [w1667]
              tunnel: w1644 -> [w1655]
              tunnel: w1641 -> [w1654]
              tunnel: [w1666] -> _ mode=indexing
              tunnel: w1640 -> [_]
              tunnel: w1639 -> [w1650]
              tunnel: [w1664] -> w1638
              tunnel: w1637 -> [w1653] mode=indexing
              shift-right: [w1665] -> w1636
              shift-left: w1642 -> [w1665]
              tunnel: [w1661] -> w1634 mode=indexing
              tunnel: w1633 -> [w1656]
              tunnel: [w1652] -> w1632 mode=indexing
              shift-right: [w1651] -> w1630
              shift-left: w1631 -> [w1651]
              tunnel: [w1649] -> w1628
              tunnel: w1627 -> [w1647]
              tunnel: w1626 -> [w1646]
              tunnel: [w1645] -> w1625
              tunnel: w1624 -> [w1645]
              n354 = Format Into String(format string=w1667, w1655, w1654, w1653, w1647, w1646) -> (resulting string=w1666:string)  [unwired: 2 in, 1 out]
              n355 = Format Into String(format string=w1656, w1655, w1654, w1653, w1647, w1646) -> (resulting string=w1659:string)  [unwired: 2 in, 1 out]
              n356 = call "Execute query.vi"("String"=w1666, "connection reference"=w1650) -> ("Table"=w1660:string[][], "connection reference 2"=w1664:T1)  [unwired: 6 in, 2 out]
              n357 = call "Execute query.vi"("String"=w1659, "connection reference"=w1650) -> ("Table"=w1657:string[][], "connection reference 2"=w1649:T1)  [unwired: 6 in, 2 out]
              n358 = Index Array(array=w1660, index (row)=0 ("disabled index (col)")) -> (element=w1662:string[])  [unwired: 1 in]
              n359 = Index Array(array=w1657, index (col)=2 ("disabled index (col)")) -> (element=w1658:string[])  [unwired: 1 in]
              n360 = Index Array(array=w1658) -> (element=w1652:string)  [unwired: 1 in]
              n361 = Index Array(array=w1662) -> (element=w1661:string)  [unwired: 1 in]
            }
            n362 = Build Array (concatenate)(w1636, w1634) -> (w1635:string[][])
            n363 = Build Array (concatenate)(w1630, w1632) -> (w1629:string[][])
          }
        }
      }
    }
    frame "ST 6" {
      n364 = case shown="\"2\"" w1679 {
        selector: w1679 -> [_ _ w1747 w1814 w1881]
        tunnel: w1678 -> [_ _ _ _ _]
        tunnel: w1677 -> [_ w1698 w1762 w1829 w1896]
        tunnel: w1676 -> [_ w1695 w1759 w1826 w1893]
        tunnel: [_ w1699 w1763 w1830 w1897] -> w1675
        tunnel: w1674 -> [w1681 w1694 w1757 w1824 w1891]
        tunnel: [w1681 w1693 w1756 w1823 w1890] -> w1673
        tunnel: w1672 -> [_ w1692 w1755 w1822 w1889]
        tunnel: [_ w1689 w1753 w1820 w1887] -> w1671
        tunnel: [_ w1688 w1752 w1819 w1886] -> w1670
        tunnel: w1669 -> [w1680 w1686 w1744 w1811 w1878]
        tunnel: [w1680 w1685 w1745 w1812 w1879] -> w1668
        frame "False", Default {
        }
        frame "ALL" {
          n365 = Concatenate Strings("select count(BREAKDOWN_STK_HOLD_ID) from " ("string"), "STATION_6_LOG_HISTORY" ("table"), "\n" ("string"), "Where year(BREAKDOWN_DATE) ='%s' and month(BREAKDOWN_DATE) = '%s' and\n BREAKDOWN_STK_HOLD_ID ='%d' and STATION_ID_CID_TRIGGER= '%s'" ("condition")) -> (w1697:string)
          n366 = Concatenate Strings("Select BREAKDOWN_IN_TIME,BREAKDOWN_OUT_TIME,DATEDIFF(MINUTE,BREAKDOWN_IN_TIME,BREAKDOWN_OUT_TIME)\nfrom STATION_6_LOG_HISTORY\n" ("string"), "Where year(BREAKDOWN_DATE) ='%s' and month(BREAKDOWN_DATE) = '%s' and\n BREAKDOWN_STK_HOLD_ID ='%d' and STATION_ID_CID_TRIGGER= '%s'" ("condition")) -> (w1691:string)
          n367 = for {
            tunnel: w1698 -> [w1721]
            tunnel: w1697 -> [w1720]
            tunnel: w1695 -> [w1718] mode=indexing
            tunnel: w1694 -> [w1717]
            tunnel: [w1716] -> w1693
            tunnel: w1692 -> [w1715]
            shift-right: [w1713] -> w1699
            shift-left: string[][] [] ("Output Array") -> [w1719]
            tunnel: w1691 -> [w1711]
            tunnel: [w1710] -> w1688
            shift-right: [w1706] -> w1689
            shift-left: string[][] [] ("Output Array") -> [w1707]
            tunnel: [w1705] -> w1685
            tunnel: w1686 -> [w1704]
            tunnel: "6" -> [w1703]
            n368 = for {
              tunnel: w1720 -> [w1743]
              tunnel: w1721 -> [w1733]
              tunnel: w1718 -> [w1732]
              tunnel: [w1742] -> _ mode=indexing
              tunnel: w1717 -> [w1730]
              tunnel: [w1740] -> w1716
              tunnel: w1715 -> [w1731] mode=indexing
              shift-right: [w1741] -> w1714
              shift-left: w1719 -> [w1741]
              tunnel: [w1736] -> w1712 mode=indexing
              tunnel: w1711 -> [w1734]
              tunnel: [w1727] -> w1710
              tunnel: [w1726] -> w1709 mode=indexing
              shift-right: [w1725] -> w1708
              shift-left: w1707 -> [w1725]
              tunnel: [w1723] -> w1705
              tunnel: w1704 -> [w1723]
              tunnel: w1703 -> [w1722]
              n369 = Format Into String(format string=w1734, w1733, w1732, w1731, w1722) -> (resulting string=w1735:string)  [unwired: 2 in, 1 out]
              n370 = Format Into String(format string=w1743, w1733, w1732, w1731, w1722) -> (resulting string=w1742:string)  [unwired: 2 in, 1 out]
              n371 = call "Execute query.vi"("String"=w1742, "connection reference"=w1730) -> ("Table"=w1739:string[][], "connection reference 2"=w1740:T1)  [unwired: 6 in, 2 out]
              n372 = call "Execute query.vi"("String"=w1735, "connection reference"=w1730) -> ("Table"=w1729:string[][], "connection reference 2"=w1727:T1)  [unwired: 6 in, 2 out]
              n373 = Index Array(array=w1739, index (row)=0 ("disabled index (col)")) -> (element=w1737:string[])  [unwired: 1 in]
              n374 = Index Array(array=w1729, index (col)=2 ("disabled index (col)")) -> (element=w1728:string[])  [unwired: 1 in]
              n375 = Index Array(array=w1728) -> (element=w1726:string)  [unwired: 1 in]
              n376 = Index Array(array=w1737) -> (element=w1736:string)  [unwired: 1 in]
            }
            n377 = Build Array (concatenate)(w1714, w1712) -> (w1713:string[][])
            n378 = Build Array (concatenate)(w1708, w1709) -> (w1706:string[][])
          }
        }
        frame "1" {
          n379 = Array Size(array=w1759) -> (size(s)=w1758:i32)
          n380 = Concatenate Strings("select count(BREAKDOWN_STK_HOLD_ID) from " ("string"), "STATION_6_LOG_HISTORY" ("table"), "\n" ("string"), "Where year(BREAKDOWN_DATE) ='%s' and month(BREAKDOWN_DATE) = '%s' and\n BREAKDOWN_STK_HOLD_ID ='%d' and STATION_ID_CID_TRIGGER= '%s'and\nSHIFT_ID='%s'" ("condition")) -> (w1761:string)
          n381 = Concatenate Strings("Select BREAKDOWN_IN_TIME,BREAKDOWN_OUT_TIME,DATEDIFF(MINUTE,BREAKDOWN_IN_TIME,BREAKDOWN_OUT_TIME)\nfrom STATION_6_LOG_HISTORY\n\n" ("string"), "Where year(BREAKDOWN_DATE) ='%s' and month(BREAKDOWN_DATE) = '%s' and\n BREAKDOWN_STK_HOLD_ID ='%d' and STATION_ID_CID_TRIGGER= '%s'and\nSHIFT_ID='%s'" ("condition")) -> (w1751:string)
          n382 = for {
            tunnel: w1762 -> [w1787]
            tunnel: w1761 -> [w1786]
            tunnel: w1759 -> [w1784] mode=indexing
            tunnel: w1758 -> [w1783]
            tunnel: w1757 -> [w1782]
            tunnel: [w1781] -> w1756
            tunnel: w1755 -> [w1780]
            shift-right: [w1778] -> w1763
            shift-left: string[][] [] ("Output Array") -> [w1785]
            tunnel: w1751 -> [w1776]
            shift-right: [w1772] -> w1753
            shift-left: string[][] [] ("Output Array") -> [w1774]
            tunnel: [w1771] -> w1752
            tunnel: "6" -> [w1770]
            tunnel: w1747 -> [w1769]
            tunnel: [w1768] -> w1745
            tunnel: w1744 -> [w1767]
            n383 = for {
              tunnel: w1786 -> [w1810]
              tunnel: w1787 -> [w1798]
              tunnel: w1784 -> [w1797]
              tunnel: [w1809] -> _ mode=indexing
              tunnel: w1783 -> [_]
              tunnel: w1782 -> [w1793]
              tunnel: [w1807] -> w1781
              tunnel: w1780 -> [w1796] mode=indexing
              shift-right: [w1808] -> w1779
              shift-left: w1785 -> [w1808]
              tunnel: [w1804] -> w1777 mode=indexing
              tunnel: w1776 -> [w1799]
              tunnel: [w1795] -> w1775 mode=indexing
              shift-right: [w1794] -> w1773
              shift-left: w1774 -> [w1794]
              tunnel: [w1792] -> w1771
              tunnel: w1770 -> [w1790]
              tunnel: w1769 -> [w1789]
              tunnel: [w1788] -> w1768
              tunnel: w1767 -> [w1788]
              n384 = Format Into String(format string=w1810, w1798, w1797, w1796, w1790, w1789) -> (resulting string=w1809:string)  [unwired: 2 in, 1 out]
              n385 = Format Into String(format string=w1799, w1798, w1797, w1796, w1790, w1789) -> (resulting string=w1802:string)  [unwired: 2 in, 1 out]
              n386 = call "Execute query.vi"("String"=w1809, "connection reference"=w1793) -> ("Table"=w1803:string[][], "connection reference 2"=w1807:T1)  [unwired: 6 in, 2 out]
              n387 = call "Execute query.vi"("String"=w1802, "connection reference"=w1793) -> ("Table"=w1800:string[][], "connection reference 2"=w1792:T1)  [unwired: 6 in, 2 out]
              n388 = Index Array(array=w1803, index (row)=0 ("disabled index (col)")) -> (element=w1805:string[])  [unwired: 1 in]
              n389 = Index Array(array=w1800, index (col)=2 ("disabled index (col)")) -> (element=w1801:string[])  [unwired: 1 in]
              n390 = Index Array(array=w1801) -> (element=w1795:string)  [unwired: 1 in]
              n391 = Index Array(array=w1805) -> (element=w1804:string)  [unwired: 1 in]
            }
            n392 = Build Array (concatenate)(w1779, w1777) -> (w1778:string[][])
            n393 = Build Array (concatenate)(w1773, w1775) -> (w1772:string[][])
          }
        }
        frame "2" {
          n394 = Array Size(array=w1826) -> (size(s)=w1825:i32)
          n395 = Concatenate Strings("select count(BREAKDOWN_STK_HOLD_ID) from " ("string"), "STATION_6_LOG_HISTORY" ("table"), "\n" ("string"), "Where year(BREAKDOWN_DATE) ='%s' and month(BREAKDOWN_DATE) = '%s' and\n BREAKDOWN_STK_HOLD_ID ='%d' and STATION_ID_CID_TRIGGER= '%s'and\nSHIFT_ID='%s'" ("condition")) -> (w1828:string)
          n396 = Concatenate Strings("Select BREAKDOWN_IN_TIME,BREAKDOWN_OUT_TIME,DATEDIFF(MINUTE,BREAKDOWN_IN_TIME,BREAKDOWN_OUT_TIME)\nfrom STATION_6_LOG_HISTORY\n\n" ("string"), "Where year(BREAKDOWN_DATE) ='%s' and month(BREAKDOWN_DATE) = '%s' and\n BREAKDOWN_STK_HOLD_ID ='%d' and STATION_ID_CID_TRIGGER= '%s'and\nSHIFT_ID='%s'" ("condition")) -> (w1818:string)
          n397 = for {
            tunnel: w1829 -> [w1854]
            tunnel: w1828 -> [w1853]
            tunnel: w1826 -> [w1851] mode=indexing
            tunnel: w1825 -> [w1850]
            tunnel: w1824 -> [w1849]
            tunnel: [w1848] -> w1823
            tunnel: w1822 -> [w1847]
            shift-right: [w1845] -> w1830
            shift-left: string[][] [] ("Output Array") -> [w1852]
            tunnel: w1818 -> [w1843]
            shift-right: [w1839] -> w1820
            shift-left: string[][] [] ("Output Array") -> [w1841]
            tunnel: [w1838] -> w1819
            tunnel: "6" -> [w1837]
            tunnel: w1814 -> [w1836]
            tunnel: [w1835] -> w1812
            tunnel: w1811 -> [w1834]
            n398 = for {
              tunnel: w1853 -> [w1877]
              tunnel: w1854 -> [w1865]
              tunnel: w1851 -> [w1864]
              tunnel: [w1876] -> _ mode=indexing
              tunnel: w1850 -> [_]
              tunnel: w1849 -> [w1860]
              tunnel: [w1874] -> w1848
              tunnel: w1847 -> [w1863] mode=indexing
              shift-right: [w1875] -> w1846
              shift-left: w1852 -> [w1875]
              tunnel: [w1871] -> w1844 mode=indexing
              tunnel: w1843 -> [w1866]
              tunnel: [w1862] -> w1842 mode=indexing
              shift-right: [w1861] -> w1840
              shift-left: w1841 -> [w1861]
              tunnel: [w1859] -> w1838
              tunnel: w1837 -> [w1857]
              tunnel: w1836 -> [w1856]
              tunnel: [w1855] -> w1835
              tunnel: w1834 -> [w1855]
              n399 = Format Into String(format string=w1877, w1865, w1864, w1863, w1857, w1856) -> (resulting string=w1876:string)  [unwired: 2 in, 1 out]
              n400 = Format Into String(format string=w1866, w1865, w1864, w1863, w1857, w1856) -> (resulting string=w1869:string)  [unwired: 2 in, 1 out]
              n401 = call "Execute query.vi"("String"=w1876, "connection reference"=w1860) -> ("Table"=w1870:string[][], "connection reference 2"=w1874:T1)  [unwired: 6 in, 2 out]
              n402 = call "Execute query.vi"("String"=w1869, "connection reference"=w1860) -> ("Table"=w1867:string[][], "connection reference 2"=w1859:T1)  [unwired: 6 in, 2 out]
              n403 = Index Array(array=w1870, index (row)=0 ("disabled index (col)")) -> (element=w1872:string[])  [unwired: 1 in]
              n404 = Index Array(array=w1867, index (col)=2 ("disabled index (col)")) -> (element=w1868:string[])  [unwired: 1 in]
              n405 = Index Array(array=w1868) -> (element=w1862:string)  [unwired: 1 in]
              n406 = Index Array(array=w1872) -> (element=w1871:string)  [unwired: 1 in]
            }
            n407 = Build Array (concatenate)(w1846, w1844) -> (w1845:string[][])
            n408 = Build Array (concatenate)(w1840, w1842) -> (w1839:string[][])
          }
        }
        frame "3" {
          n409 = Array Size(array=w1893) -> (size(s)=w1892:i32)
          n410 = Concatenate Strings("select count(BREAKDOWN_STK_HOLD_ID) from " ("string"), "STATION_6_LOG_HISTORY" ("table"), "\n" ("string"), "Where year(BREAKDOWN_DATE) ='%s' and month(BREAKDOWN_DATE) = '%s' and\n BREAKDOWN_STK_HOLD_ID ='%d' and STATION_ID_CID_TRIGGER= '%s'and\nSHIFT_ID='%s'" ("condition")) -> (w1895:string)
          n411 = Concatenate Strings("Select BREAKDOWN_IN_TIME,BREAKDOWN_OUT_TIME,DATEDIFF(MINUTE,BREAKDOWN_IN_TIME,BREAKDOWN_OUT_TIME)\nfrom STATION_6_LOG_HISTORY\n\n" ("string"), "Where year(BREAKDOWN_DATE) ='%s' and month(BREAKDOWN_DATE) = '%s' and\n BREAKDOWN_STK_HOLD_ID ='%d' and STATION_ID_CID_TRIGGER= '%s'and\nSHIFT_ID='%s'" ("condition")) -> (w1885:string)
          n412 = for {
            tunnel: w1896 -> [w1921]
            tunnel: w1895 -> [w1920]
            tunnel: w1893 -> [w1918] mode=indexing
            tunnel: w1892 -> [w1917]
            tunnel: w1891 -> [w1916]
            tunnel: [w1915] -> w1890
            tunnel: w1889 -> [w1914]
            shift-right: [w1912] -> w1897
            shift-left: string[][] [] ("Output Array") -> [w1919]
            tunnel: w1885 -> [w1910]
            shift-right: [w1906] -> w1887
            shift-left: string[][] [] ("Output Array") -> [w1908]
            tunnel: [w1905] -> w1886
            tunnel: "6" -> [w1904]
            tunnel: w1881 -> [w1903]
            tunnel: [w1902] -> w1879
            tunnel: w1878 -> [w1901]
            n413 = for {
              tunnel: w1920 -> [w1944]
              tunnel: w1921 -> [w1932]
              tunnel: w1918 -> [w1931]
              tunnel: [w1943] -> _ mode=indexing
              tunnel: w1917 -> [_]
              tunnel: w1916 -> [w1927]
              tunnel: [w1941] -> w1915
              tunnel: w1914 -> [w1930] mode=indexing
              shift-right: [w1942] -> w1913
              shift-left: w1919 -> [w1942]
              tunnel: [w1938] -> w1911 mode=indexing
              tunnel: w1910 -> [w1933]
              tunnel: [w1929] -> w1909 mode=indexing
              shift-right: [w1928] -> w1907
              shift-left: w1908 -> [w1928]
              tunnel: [w1926] -> w1905
              tunnel: w1904 -> [w1924]
              tunnel: w1903 -> [w1923]
              tunnel: [w1922] -> w1902
              tunnel: w1901 -> [w1922]
              n414 = Format Into String(format string=w1944, w1932, w1931, w1930, w1924, w1923) -> (resulting string=w1943:string)  [unwired: 2 in, 1 out]
              n415 = Format Into String(format string=w1933, w1932, w1931, w1930, w1924, w1923) -> (resulting string=w1936:string)  [unwired: 2 in, 1 out]
              n416 = call "Execute query.vi"("String"=w1943, "connection reference"=w1927) -> ("Table"=w1937:string[][], "connection reference 2"=w1941:T1)  [unwired: 6 in, 2 out]
              n417 = call "Execute query.vi"("String"=w1936, "connection reference"=w1927) -> ("Table"=w1934:string[][], "connection reference 2"=w1926:T1)  [unwired: 6 in, 2 out]
              n418 = Index Array(array=w1937, index (row)=0 ("disabled index (col)")) -> (element=w1939:string[])  [unwired: 1 in]
              n419 = Index Array(array=w1934, index (col)=2 ("disabled index (col)")) -> (element=w1935:string[])  [unwired: 1 in]
              n420 = Index Array(array=w1935) -> (element=w1929:string)  [unwired: 1 in]
              n421 = Index Array(array=w1939) -> (element=w1938:string)  [unwired: 1 in]
            }
            n422 = Build Array (concatenate)(w1913, w1911) -> (w1912:string[][])
            n423 = Build Array (concatenate)(w1907, w1909) -> (w1906:string[][])
          }
        }
      }
    }
  }
  "BD Count" <- w9
  "connection reference 2" <- w7
  "error out" <- w3
  "Duration count" <- w5
